vi "RFmx_MeasTest_Analysis.vi"(8 "error in (no error)":errorcluster, 11 "Message_Queues":T3) -> (0 "error out":errorcluster)   [LabVIEW 2014]
uses:
  02_Controls/Message_Queues.ctl
  02_Controls/Message_Data_Ctl.ctl
  15_DataManagement/Analysis_Parameters.ctl
  SubVIs/RFmx_An_Disp_Ctrl.ctl
panel:
  in  "Tab Control":T1=enum."CCDF"
  out "ACP":cluster{"x0":dbl, "dx":dbl, "y":sgl[]}[](graph)=[{"x0"=1134999754.066313, "dx"=998.2196003401557, "y"=array[30055 elements]}, {"x0"=0.0, "dx"=0.0, "y"=[]}, {"x0"=0.0, "dx"=0.0, "y"=[]}, {"x0"=0.0, "dx"=0.0, "y"=[]}, {"x0"=1134999754.066313, "dx"=998.2196003401557, "y"=array[30055 elements]}]
  out "ACP_Data":dbl[](array[numeric])=[750000.0, -20.734813690185547, 53.66733169555664, 3.519465684890747] format="%#_6p"
  out "CHP":cluster{"x0":dbl, "dx":dbl, "y":sgl[]}[](graph)=[{"x0"=1134999754.066313, "dx"=998.2196003401557, "y"=array[30055 elements]}, {"x0"=1134999754.066313, "dx"=998.2196003401557, "y"=array[30055 elements]}]
  out "OBW":cluster{"x0":dbl, "dx":dbl, "y":sgl[]}[](graph)=[{"x0"=1134999754.066313, "dx"=998.2196003401557, "y"=array[30055 elements]}, {"x0"=1134999754.066313, "dx"=998.2196003401557, "y"=array[30055 elements]}]
  out "TXP_PwrTrace":cluster{"x0":dbl, "dx":dbl, "y":sgl[]}(graph)={"x0"=-4.98745570667522e-12, "dx"=1.333333333320651e-05, "y"=[-70.1271, -70.102455, -70.09967, -70.138626, -70.2021, -70.25555, -70.28413, -70.29169, -70.28087, -70.246735, -70.18414, -70.09316, -69.98076, -69.8681, -69.79553, -69.79967, -69.875374, -69.97399, -70.04578, -70.074875, -70.0764, -70.07251, -70.0786, -70.099106, -70.12221, -70.11699, -70.06154, -69.987854, -69.97353, -70.07697, -70.28213, -70.49838, -70.619514, -70.604355, -70.50262, -70.399666, -70.34924, -70.354, -70.3841, -70.40493, -70.39727, -70.36025, -70.31259, -70.28346, -70.279724, -70.2837, -70.28102, -70.27398, -70.273705, -70.28955, -70.32246, -70.36373, -70.40005, -70.4229, -70.43052, -70.42366, -70.40363, -70.3778, -70.36408, -70.38452, -70.44807, -70.549355, -70.66728, -70.747925, -70.71708, -70.54683, -70.28816, -70.03155, -69.85307, -69.78543, -69.80181, -69.82049, -69.76297, -69.637566, -69.54464, -69.58453, -69.76692, -70.01199, -70.22523, -70.36874, -70.46258, -70.54471, -70.628296, -70.689095, -70.6958, -70.644844, -70.56589, -70.49992, -70.466835, -70.457146, -70.45056, -70.43114, -70.392235, -70.34338, -70.30397, -70.285736, -70.28102, -70.272095, -70.249214, -70.227776, -70.24491, -70.31819, -70.41253, -70.4785, -70.50577, -70.51349, -70.51906, -70.53742, -70.59497, -70.73529, -71.00162, -71.38568, -71.789246, -72.070625, -72.15951, -72.077644, -71.88744, -71.65048, -71.38336, -71.0968, -70.85372, -70.712296, -70.648, -70.59169, -70.51985, -70.46071, -70.434654, -70.42709, -70.41435, -70.38291, -70.33717, -70.294846, -70.267975, -70.25562, -70.250694, -70.24638, -70.23686, -70.21681, -70.185425, -70.152855, -70.13762, -70.14813, -70.1704, -70.18109, -70.168976, -70.14167, -70.11527, -70.09345, -70.06084, -70.00988, -69.97303, -70.01334, -70.162346, -70.36518, -70.51255, -70.52762, -70.410835, -70.21521, -70.005104, -69.83721, -69.753, -69.76635, -69.85591, -69.97935, -70.09232, -70.160034, -70.176285, -70.17383, -70.195854, -70.25506, -70.34203, -70.46222, -70.63041, -70.81692, -70.9472, -70.98923, -71.01785, -71.1728, -71.53291, -72.01664, -72.406296, -72.52623, -72.40028, -72.1804, -71.96133, -71.74775, -71.57884, -71.5427, -71.664444, -71.86329, -72.009705, -72.022285, -71.9312, -71.82318, -71.7381, -71.65193, -71.51254, -71.2917, -71.03287, -70.83856, -70.78675, -70.868, -71.01887, -71.202896, -71.43712, -71.73827, -72.08321, -72.42074, -72.6703, -72.712105, -72.46677, -72.00842, -71.53421, -71.24306, -71.24765, -71.53821, -71.9796, -72.376366, -72.59654, -72.640526, -72.58551, -72.46033, -72.21592, -71.82655, -71.36928, -70.96878, -70.70235, -70.57518, -70.55464, -70.60321, -70.671196, -70.69574, -70.64515, -70.55917, -70.52155, -70.60362, -70.83718, -71.20136, -71.60672, -71.91493, -72.01895, -71.92462, -71.7453, -71.60187, -71.52983, -71.46005, -71.2856, -70.983475, -70.640854, -70.35246, -70.154205, -70.0494, -70.03544, -70.094894, -70.19584, -70.31638, -70.43914, -70.52042, -70.50131, -70.36992, -70.1966, -70.08757, -70.114914, -70.280266, -70.516754, -70.73874, -70.904396, -71.013405, -71.041016, -70.93407, -70.69386, -70.42141, -70.24169, -70.20023, -70.24776, -70.31064, -70.36012, -70.392685, -70.38757, -70.330055, -70.24892, -70.188736, -70.15334, -70.11064, -70.04098, -69.960236, -69.90947, -69.93629, -70.0791, -70.33356, -70.624886, -70.83586, -70.89375, -70.814514, -70.66997, -70.5526, -70.55675, -70.7309, -71.01462, -71.242516, -71.27896, -71.148766, -70.98232, -70.870804, -70.81653, -70.76519, -70.67791, -70.57681, -70.49742, -70.42339, -70.31814, -70.21381, -70.21159, -70.38383, -70.68958, -70.97363, -71.07428, -70.959236, -70.73489, -70.52688, -70.393105, -70.333824, -70.32502, -70.33476, -70.33452, -70.309326, -70.263794, -70.22499, -70.22239, -70.25476, -70.29094, -70.30613, -70.300125, -70.29144, -70.30344, -70.35219, -70.433464, -70.51426, -70.549385, -70.519104, -70.44781, -70.38268, -70.35341, -70.35752, -70.38461, -70.448654, -70.590775, -70.83775, -71.13816, -71.36328, -71.40347, -71.26845, -71.06155, -70.86465, -70.68394, -70.50064, -70.32482, -70.18509, -70.09302, -70.034256, -69.9907, -69.96237, -69.96383, -70.00722, -70.1008, -70.25221, -70.43503, -70.563286, -70.54413, -70.37306, -70.14535, -69.97606, -69.93775, -70.051865, -70.298836, -70.63075, -70.96844, -71.191925, -71.19785, -71.00357, -70.74416, -70.549095, -70.45745, -70.44101, -70.46208, -70.487526, -70.48328, -70.42944, -70.336716, -70.23764, -70.16715, -70.15245, -70.20595, -70.33126, -70.523056, -70.75548, -70.97542, -71.127914, -71.20036, -71.23254, -71.283714, -71.37482, -71.45885, -71.4582, -71.33722, -71.131905, -70.918884, -70.764725, -70.68758, -70.66344, -70.66629, -70.69003, -70.72007, -70.712395, -70.63426, -70.510025, -70.401115, -70.349625, -70.3556, -70.38955, -70.41931, -70.42943, -70.419876, -70.392715, -70.3439, -70.26482, -70.16419, -70.09059, -70.11067, -70.25772, -70.50903, -70.78793, -70.98342, -71.03065, -70.987206, -70.957726, -70.95307, -70.904144, -70.802505, -70.74672, -70.8326, -71.03998, -71.23038, -71.261185, -71.11531, -70.89604, -70.718994, -70.64278, -70.67297, -70.77545, -70.88165, -70.92553, -70.91127, -70.90201, -70.920334, -70.9097, -70.81249, -70.642, -70.460976, -70.31799, -70.22179, -70.16339, -70.14114, -70.153564, -70.18681, -70.22244, -70.25476, -70.29089, -70.336296, -70.38193, -70.41022, -70.41077, -70.38516, -70.348206, -70.32399, -70.325325, -70.34256, -70.36334, -70.393364, -70.460625, -70.59186, -70.7767, -70.9539, -71.04438, -71.00727, -70.867874, -70.70291, -70.59369, -70.58453, -70.66925, -70.80333, -70.94123, -71.07266, -71.21135, -71.34671, -71.45471, -71.549774, -71.671684, -71.794785, -71.811935, -71.66149, -71.427444, -71.25798, -71.22795, -71.29315, -71.352036, -71.342224, -71.270226, -71.180084, -71.12189, -71.12526, -71.16607, -71.166954, -71.058426, -70.8422, -70.58765, -70.36951, -70.23198, -70.196075, -70.2832, -70.51522, -70.87754, -71.28055, -71.57588, -71.675446, -71.65345, -71.67442, -71.82185, -72.03004, -72.15217, -72.0683, -71.75293, -71.28349, -70.800285, -70.4402, -70.29247, -70.386894, -70.681244, -71.05052, -71.34525, -71.526794, -71.67786, -71.83254, -71.921036, -71.908615, -71.85493, -71.82098, -71.81082, -71.788025, -71.70886, -71.56084, -71.38074, -71.21522, -71.06775, -70.89776, -70.67848, -70.443886, -70.26495, -70.18929, -70.22381, -70.34598, -70.49758, -70.59422, -70.58327, -70.492256, -70.39598, -70.34745, -70.350945, -70.376526, -70.388756, -70.3667, -70.309906, -70.24661, -70.21888, -70.239075, -70.283875, -70.32356, -70.34142, -70.336464, -70.32062, -70.31242, -70.32254, -70.34507, -70.37217, -70.412254, -70.48494, -70.5921, -70.68931, -70.716415, -70.67915, -70.666595, -70.74049, -70.857124, -70.93891, -70.9912, -71.096535, -71.29889, -71.51818, -71.59646, -71.452415, -71.16241, -70.88185, -70.715324, -70.66288, -70.66028, -70.64644, -70.606415, -70.55378, -70.50803, -70.49969, -70.54775, -70.62311, -70.68454, -70.736206, -70.801315, -70.87974, -70.95877, -71.03975, -71.11876, -71.166214, -71.14653, -71.04972, -70.898445, -70.7247, -70.55195, -70.39522, -70.260086, -70.15135, -70.08678, -70.08174, -70.123795, -70.18848, -70.26684, -70.3716, -70.513985, -70.674736, -70.808716, -70.881485, -70.885155, -70.82721, -70.73247, -70.65466, -70.64117, -70.676765, -70.68882, -70.624115, -70.50197, -70.38329, -70.30879, -70.28491, -70.30879, -70.38329, -70.50113, -70.6197, -70.67169, -70.624115, -70.51857, -70.43616, -70.43359, -70.50927, -70.6081, -70.66765, -70.68427, -70.72201, -70.82337, -70.94429, -71.00236, -70.96122, -70.84161, -70.70359, -70.64045, -70.72783, -70.940865, -71.137505, -71.172806, -71.041145, -70.85834, -70.719444, -70.62562, -70.53578, -70.43355, -70.338165, -70.27004, -70.235825, -70.242905, -70.30614, -70.429855, -70.5876, -70.72852, -70.80606, -70.789406, -70.65997, -70.43023, -70.17071, -69.97722, -69.89921, -69.91674, -69.98164, -70.059425, -70.140335, -70.22925, -70.334366, -70.46442, -70.61354, -70.73899, -70.77561, -70.70575, -70.59821, -70.559265, -70.65948, -70.90869, -71.270645, -71.67924, -72.03883, -72.237366, -72.20009, -71.96115, -71.65437, -71.408066, -71.2635, -71.18208, -71.09467, -70.94478, -70.727875, -70.51102, -70.37953, -70.36407, -70.437836, -70.550835, -70.63729, -70.63367, -70.53299, -70.404144, -70.337685, -70.38474, -70.543526, -70.75984, -70.94081, -71.0143, -70.999954, -70.99277, -71.043396, -71.07776, -70.98049, -70.75311, -70.525215, -70.41042, -70.41771, -70.501976, -70.62645]}
  out "CCDF_PwrTrace":cluster{"x0":dbl, "dx":dbl, "y":sgl[]}[](graph)=[{"x0"=0.0, "dx"=0.05, "y"=[53.66733, 52.4644, 51.195732, 49.906933, 48.5928, 47.24, 45.878, 44.492535, 43.0708, 41.638268, 40.190933, 38.7444, 37.3052, 35.848, 34.410667, 32.9784, 31.523867, 30.067734, 28.628933, 27.1972, 25.780666, 24.380667, 22.984533, 21.613333, 20.296667, 19.015066, 17.751333, 16.544134, 15.362267, 14.232, 13.1368, 12.0996, 11.079866, 10.1244, 9.173734, 8.2868, 7.4492, 6.670533, 5.9525332, 5.295067, 4.6957335, 4.153333, 3.6621332, 3.2249334, 2.8288, 2.4806666, 2.1506667, 1.8712, 1.6233333, 1.4028, 1.2012, 1.028, 0.8810667, 0.74453336, 0.6264, 0.5182667, 0.4148, 0.32906666, 0.2516, 0.18853334, 0.14026667, 0.0992, 0.06893333, 0.048933335, 0.031466667, 0.019066667, 0.010533334, 0.0052, 0.0028, 0.0014666667, 0.0004, 0.0, 0.0, 0.0, 0.0, 0.0, 0.0, 0.0, 0.0, 0.0, 0.0, 0.0, 0.0, 0.0, 0.0, 0.0, 0.0, 0.0, 0.0, 0.0, 0.0, 0.0, 0.0, 0.0, 0.0, 0.0, 0.0, 0.0, 0.0, 0.0, 0.0, 0.0, 0.0, 0.0, 0.0, 0.0, 0.0, 0.0, 0.0, 0.0, 0.0, 0.0, 0.0, 0.0, 0.0, 0.0, 0.0, 0.0, 0.0, 0.0, 0.0, 0.0, 0.0, 0.0, 0.0, 0.0, 0.0, 0.0, 0.0, 0.0, 0.0, 0.0, 0.0, 0.0, 0.0, 0.0, 0.0, 0.0, 0.0, 0.0, 0.0, 0.0, 0.0, 0.0, 0.0, 0.0, 0.0, 0.0, 0.0, 0.0, 0.0, 0.0, 0.0, 0.0, 0.0, 0.0, 0.0, 0.0, 0.0, 0.0, 0.0, 0.0, 0.0, 0.0, 0.0, 0.0, 0.0, 0.0, 0.0, 0.0, 0.0, 0.0, 0.0, 0.0, 0.0, 0.0, 0.0, 0.0, 0.0, 0.0, 0.0, 0.0, 0.0, 0.0, 0.0, 0.0, 0.0, 0.0, 0.0, 0.0, 0.0, 0.0, 0.0, 0.0, 0.0, 0.0, 0.0, 0.0, 0.0, 0.0, 0.0, 0.0, 0.0, 0.0, 0.0, 0.0, 0.0, 0.0, 0.0, 0.0, 0.0, 0.0, 0.0, 0.0, 0.0, 0.0, 0.0, 0.0, 0.0, 0.0, 0.0, 0.0, 0.0, 0.0, 0.0, 0.0, 0.0, 0.0, 0.0, 0.0, 0.0, 0.0, 0.0, 0.0, 0.0, 0.0, 0.0, 0.0, 0.0, 0.0, 0.0, 0.0, 0.0, 0.0, 0.0, 0.0, 0.0, 0.0, 0.0, 0.0, 0.0, 0.0, 0.0, 0.0, 0.0, 0.0, 0.0, 0.0, 0.0, 0.0, 0.0, 0.0, 0.0, 0.0, 0.0, 0.0, 0.0, 0.0, 0.0, 0.0, 0.0, 0.0, 0.0, 0.0, 0.0, 0.0, 0.0, 0.0, 0.0, 0.0, 0.0, 0.0, 0.0, 0.0, 0.0, 0.0, 0.0, 0.0, 0.0, 0.0, 0.0, 0.0, 0.0, 0.0, 0.0, 0.0, 0.0, 0.0, 0.0, 0.0, 0.0, 0.0, 0.0, 0.0, 0.0, 0.0, 0.0, 0.0, 0.0, 0.0, 0.0, 0.0, 0.0, 0.0, 0.0, 0.0, 0.0, 0.0, 0.0, 0.0, 0.0, 0.0, 0.0, 0.0, 0.0, 0.0, 0.0, 0.0, 0.0, 0.0, 0.0, 0.0, 0.0, 0.0, 0.0, 0.0, 0.0, 0.0, 0.0, 0.0, 0.0, 0.0, 0.0, 0.0, 0.0, 0.0, 0.0, 0.0, 0.0, 0.0, 0.0, 0.0, 0.0, 0.0, 0.0, 0.0, 0.0, 0.0, 0.0, 0.0, 0.0, 0.0, 0.0, 0.0, 0.0, 0.0, 0.0, 0.0, 0.0, 0.0, 0.0, 0.0, 0.0, 0.0, 0.0, 0.0, 0.0, 0.0, 0.0, 0.0, 0.0, 0.0, 0.0, 0.0, 0.0, 0.0, 0.0, 0.0, 0.0, 0.0, 0.0, 0.0, 0.0, 0.0, 0.0, 0.0, 0.0, 0.0, 0.0, 0.0]}, {"x0"=0.0, "dx"=0.05, "y"=[36.787945, 36.364418, 35.940945, 35.51759, 35.094402, 34.671444, 34.24878, 33.826458, 33.404545, 32.9831, 32.562187, 32.141865, 31.722195, 31.30324, 30.885061, 30.467726, 30.051294, 29.635832, 29.221403, 28.808071, 28.3959, 27.984957, 27.575306, 27.167011, 26.76014, 26.354755, 25.950926, 25.548716, 25.14819, 24.749414, 24.352455, 23.957375, 23.564243, 23.17312, 22.784075, 22.39717, 22.012466, 21.630032, 21.24993, 20.872221, 20.49697, 20.124235, 19.75408, 19.386568, 19.021753, 18.6597, 18.300467, 17.944107, 17.590683, 17.240246, 16.892855, 16.548563, 16.207422, 15.869487, 15.534806, 15.20343, 14.875409, 14.55079, 14.229618, 13.91194, 13.597798, 13.287235, 12.980292, 12.677009, 12.377422, 12.08157, 11.789486, 11.501204, 11.216754, 10.936168, 10.659473, 10.386697, 10.117864, 9.852996, 9.592114, 9.33524, 9.082389, 8.833577, 8.5888195, 8.348126, 8.111507, 7.8789725, 7.650526, 7.4261727, 7.205915, 6.9897523, 6.7776837, 6.5697045, 6.36581, 6.165992, 5.9702406, 5.778545, 5.590891, 5.4072638, 5.2276454, 5.052017, 4.8803573, 4.7126436, 4.5488515, 4.3889537, 4.232922, 4.0807266, 3.9323359, 3.7877162, 3.6468325, 3.509648, 3.376125, 3.2462234, 3.1199024, 2.997119, 2.8778293, 2.7619884, 2.6495495, 2.540465, 2.4346862, 2.3321629, 2.2328444, 2.1366782, 2.0436118, 1.9535915, 1.8665625, 1.7824696, 1.701257, 1.6228681, 1.5472456, 1.4743322, 1.4040698, 1.3364, 1.2712642, 1.2086037, 1.1483593, 1.0904721, 1.0348829, 0.98153263, 0.9303623, 0.881313, 0.83432627, 0.78934366, 0.7463072, 0.7051592, 0.6658425, 0.62830037, 0.5924767, 0.558316, 0.52576315, 0.49476406, 0.46526518, 0.43721372, 0.4105578, 0.3852463, 0.36122903, 0.3384567, 0.31688094, 0.29645437, 0.2771306, 0.2588643, 0.24161115, 0.22532786, 0.20997226, 0.19550326, 0.18188089, 0.16906624, 0.15702157, 0.14571023, 0.13509673, 0.12514666, 0.11582677, 0.10710493, 0.09895011, 0.09133239, 0.084222965, 0.077594094, 0.071419135, 0.065672494, 0.060329612, 0.055366978, 0.050762083, 0.04649341, 0.042540405, 0.038883466, 0.03550392, 0.032383993, 0.029506788, 0.02685626, 0.0244172, 0.02217519, 0.020116596, 0.018228529, 0.016498832, 0.0149160335, 0.013469341, 0.012148602, 0.010944282, 0.009847437, 0.008849691, 0.007943204, 0.007120654, 0.0063752076, 0.0057004965, 0.005090594, 0.004539993, 0.004043582, 0.0035966237, 0.003194734, 0.0028338607, 0.0025102647, 0.0022205, 0.0019613956, 0.0017300382, 0.0015237544, 0.0013400955, 0.0011768217, 0.0010318871, 0.0009034264, 0.0007897411, 0.0006892875, 0.0006006644, 0.0005226023, 0.0004539527, 0.00039367852, 0.0003408446, 0.00029460926, 0.00025421623, 0.00021898713, 0.00018831449, 0.00016165532, 0.00013852515, 0.00011849246, 0.000101173624, 8.622819e-05, 7.3354604e-05, 6.228628e-05, 5.2787957e-05, 4.4652443e-05, 3.7697617e-05, 3.1763702e-05, 2.6710808e-05, 2.2416698e-05, 1.8774781e-05, 1.5692298e-05, 1.3088694e-05, 1.08941595e-05, 9.048326e-06, 7.4991e-06, 6.201627e-06, 5.1173697e-06, 4.2132915e-06, 3.461136e-06, 2.836788e-06, 2.3197156e-06, 1.8924771e-06, 1.5402914e-06, 1.250661e-06, 1.0130451e-06, 8.185747e-07, 6.598055e-07, 5.3050474e-07, 4.254668e-07, 3.4035529e-07, 2.7156693e-07, 2.1611548e-07, 1.7153243e-07, 1.357828e-07, 1.0719338e-07, 8.439218e-08, 6.62573e-08, 5.1873865e-08, 4.0497927e-08, 3.1526227e-08, 2.4471005e-08, 1.8939026e-08, 1.461419e-08, 1.1243155e-08, 8.623487e-09, 6.593919e-09, 5.0263744e-09, 3.8194514e-09, 2.8931189e-09, 2.1844124e-09, 1.6439551e-09, 1.2331498e-09, 9.2192537e-10, 6.8693073e-10, 5.1009436e-10, 3.7747766e-10, 2.7836708e-10, 2.045563e-10, 1.497816e-10, 1.09279e-10, 7.943822e-11, 5.753319e-11, 4.151308e-11, 2.984079e-11, 2.136857e-11, 1.5242675e-11, 1.08304875e-11, 7.6650734e-12, 5.4031393e-12, 3.7933025e-12, 2.6522215e-12, 1.8467268e-12, 1.2804867e-12, 8.8410946e-13, 6.0781897e-13, 4.1606207e-13, 2.8355402e-13, 1.9239123e-13, 1.2995236e-13, 8.737957e-14, 5.848435e-14, 3.896281e-14, 2.5835592e-14, 1.7049845e-14, 1.1197791e-14, 7.318634e-15, 4.7598025e-15, 3.0802383e-15, 1.9833124e-15, 1.2705274e-15, 8.097247e-16, 5.133638e-16, 3.2375868e-16, 2.0309505e-16, 1.267162e-16, 7.86308e-17, 4.852366e-17, 2.9777407e-17, 1.8170405e-17, 1.10244845e-17, 6.650268e-18, 3.9882104e-18, 2.3776376e-18, 1.4090037e-18, 8.2994133e-19, 4.8587095e-19, 2.8268445e-19, 1.6344032e-19, 9.389906e-20, 5.36014e-20, 3.039986e-20, 1.7128329e-20, 9.586792e-21, 5.329827e-21, 2.94307e-21, 1.6139929e-21, 8.789851e-22, 4.753412e-22, 2.552336e-22, 1.3606395e-22, 7.200868e-23, 3.7829146e-23, 1.972564e-23, 1.0208479e-23, 5.242983e-24, 2.6720525e-24, 1.3512067e-24, 6.779063e-25, 3.3740296e-25, 1.6657864e-25, 8.157184e-26, 3.9616006e-26, 1.9079589e-26, 9.111568e-27, 4.314202e-27, 2.0251076e-27, 9.423071e-28, 4.345997e-28, 1.9865274e-28, 8.998346e-29, 4.0387624e-29, 1.7959954e-29, 7.9120106e-30, 3.452598e-30, 1.4922271e-30, 6.387123e-31, 2.707125e-31, 1.1360423e-31, 4.7196953e-32, 1.9409576e-32, 7.900411e-33, 3.182461e-33, 1.2685392e-33, 5.00287e-34, 1.9518905e-34, 7.532834e-35, 2.8752345e-35, 1.08528714e-35, 4.0505728e-36, 1.4946238e-36, 5.451721e-37, 1.965457e-37, 7.002659e-38, 2.4653156e-38, 8.574959e-39, 2.946325e-39, 9.99901e-40, 3.35119e-40, 1.10903e-40, 3.62348e-41, 1.16868e-41]}]
  out "CCDF_Data":dbl[](array[numeric])=[750000.0, -20.734813690185547, 53.66733333333333, 3.519465684890747] format="%#_6p"
  out "Spectrum":cluster{"x0":dbl, "dx":dbl, "y":sgl[]}(graph)={"x0"=-4.98745570667522e-12, "dx"=1.333333333320651e-05, "y"=[-70.1271, -70.102455, -70.09967, -70.138626, -70.2021, -70.25555, -70.28413, -70.29169, -70.28087, -70.246735, -70.18414, -70.09316, -69.98076, -69.8681, -69.79553, -69.79967, -69.875374, -69.97399, -70.04578, -70.074875, -70.0764, -70.07251, -70.0786, -70.099106, -70.12221, -70.11699, -70.06154, -69.987854, -69.97353, -70.07697, -70.28213, -70.49838, -70.619514, -70.604355, -70.50262, -70.399666, -70.34924, -70.354, -70.3841, -70.40493, -70.39727, -70.36025, -70.31259, -70.28346, -70.279724, -70.2837, -70.28102, -70.27398, -70.273705, -70.28955, -70.32246, -70.36373, -70.40005, -70.4229, -70.43052, -70.42366, -70.40363, -70.3778, -70.36408, -70.38452, -70.44807, -70.549355, -70.66728, -70.747925, -70.71708, -70.54683, -70.28816, -70.03155, -69.85307, -69.78543, -69.80181, -69.82049, -69.76297, -69.637566, -69.54464, -69.58453, -69.76692, -70.01199, -70.22523, -70.36874, -70.46258, -70.54471, -70.628296, -70.689095, -70.6958, -70.644844, -70.56589, -70.49992, -70.466835, -70.457146, -70.45056, -70.43114, -70.392235, -70.34338, -70.30397, -70.285736, -70.28102, -70.272095, -70.249214, -70.227776, -70.24491, -70.31819, -70.41253, -70.4785, -70.50577, -70.51349, -70.51906, -70.53742, -70.59497, -70.73529, -71.00162, -71.38568, -71.789246, -72.070625, -72.15951, -72.077644, -71.88744, -71.65048, -71.38336, -71.0968, -70.85372, -70.712296, -70.648, -70.59169, -70.51985, -70.46071, -70.434654, -70.42709, -70.41435, -70.38291, -70.33717, -70.294846, -70.267975, -70.25562, -70.250694, -70.24638, -70.23686, -70.21681, -70.185425, -70.152855, -70.13762, -70.14813, -70.1704, -70.18109, -70.168976, -70.14167, -70.11527, -70.09345, -70.06084, -70.00988, -69.97303, -70.01334, -70.162346, -70.36518, -70.51255, -70.52762, -70.410835, -70.21521, -70.005104, -69.83721, -69.753, -69.76635, -69.85591, -69.97935, -70.09232, -70.160034, -70.176285, -70.17383, -70.195854, -70.25506, -70.34203, -70.46222, -70.63041, -70.81692, -70.9472, -70.98923, -71.01785, -71.1728, -71.53291, -72.01664, -72.406296, -72.52623, -72.40028, -72.1804, -71.96133, -71.74775, -71.57884, -71.5427, -71.664444, -71.86329, -72.009705, -72.022285, -71.9312, -71.82318, -71.7381, -71.65193, -71.51254, -71.2917, -71.03287, -70.83856, -70.78675, -70.868, -71.01887, -71.202896, -71.43712, -71.73827, -72.08321, -72.42074, -72.6703, -72.712105, -72.46677, -72.00842, -71.53421, -71.24306, -71.24765, -71.53821, -71.9796, -72.376366, -72.59654, -72.640526, -72.58551, -72.46033, -72.21592, -71.82655, -71.36928, -70.96878, -70.70235, -70.57518, -70.55464, -70.60321, -70.671196, -70.69574, -70.64515, -70.55917, -70.52155, -70.60362, -70.83718, -71.20136, -71.60672, -71.91493, -72.01895, -71.92462, -71.7453, -71.60187, -71.52983, -71.46005, -71.2856, -70.983475, -70.640854, -70.35246, -70.154205, -70.0494, -70.03544, -70.094894, -70.19584, -70.31638, -70.43914, -70.52042, -70.50131, -70.36992, -70.1966, -70.08757, -70.114914, -70.280266, -70.516754, -70.73874, -70.904396, -71.013405, -71.041016, -70.93407, -70.69386, -70.42141, -70.24169, -70.20023, -70.24776, -70.31064, -70.36012, -70.392685, -70.38757, -70.330055, -70.24892, -70.188736, -70.15334, -70.11064, -70.04098, -69.960236, -69.90947, -69.93629, -70.0791, -70.33356, -70.624886, -70.83586, -70.89375, -70.814514, -70.66997, -70.5526, -70.55675, -70.7309, -71.01462, -71.242516, -71.27896, -71.148766, -70.98232, -70.870804, -70.81653, -70.76519, -70.67791, -70.57681, -70.49742, -70.42339, -70.31814, -70.21381, -70.21159, -70.38383, -70.68958, -70.97363, -71.07428, -70.959236, -70.73489, -70.52688, -70.393105, -70.333824, -70.32502, -70.33476, -70.33452, -70.309326, -70.263794, -70.22499, -70.22239, -70.25476, -70.29094, -70.30613, -70.300125, -70.29144, -70.30344, -70.35219, -70.433464, -70.51426, -70.549385, -70.519104, -70.44781, -70.38268, -70.35341, -70.35752, -70.38461, -70.448654, -70.590775, -70.83775, -71.13816, -71.36328, -71.40347, -71.26845, -71.06155, -70.86465, -70.68394, -70.50064, -70.32482, -70.18509, -70.09302, -70.034256, -69.9907, -69.96237, -69.96383, -70.00722, -70.1008, -70.25221, -70.43503, -70.563286, -70.54413, -70.37306, -70.14535, -69.97606, -69.93775, -70.051865, -70.298836, -70.63075, -70.96844, -71.191925, -71.19785, -71.00357, -70.74416, -70.549095, -70.45745, -70.44101, -70.46208, -70.487526, -70.48328, -70.42944, -70.336716, -70.23764, -70.16715, -70.15245, -70.20595, -70.33126, -70.523056, -70.75548, -70.97542, -71.127914, -71.20036, -71.23254, -71.283714, -71.37482, -71.45885, -71.4582, -71.33722, -71.131905, -70.918884, -70.764725, -70.68758, -70.66344, -70.66629, -70.69003, -70.72007, -70.712395, -70.63426, -70.510025, -70.401115, -70.349625, -70.3556, -70.38955, -70.41931, -70.42943, -70.419876, -70.392715, -70.3439, -70.26482, -70.16419, -70.09059, -70.11067, -70.25772, -70.50903, -70.78793, -70.98342, -71.03065, -70.987206, -70.957726, -70.95307, -70.904144, -70.802505, -70.74672, -70.8326, -71.03998, -71.23038, -71.261185, -71.11531, -70.89604, -70.718994, -70.64278, -70.67297, -70.77545, -70.88165, -70.92553, -70.91127, -70.90201, -70.920334, -70.9097, -70.81249, -70.642, -70.460976, -70.31799, -70.22179, -70.16339, -70.14114, -70.153564, -70.18681, -70.22244, -70.25476, -70.29089, -70.336296, -70.38193, -70.41022, -70.41077, -70.38516, -70.348206, -70.32399, -70.325325, -70.34256, -70.36334, -70.393364, -70.460625, -70.59186, -70.7767, -70.9539, -71.04438, -71.00727, -70.867874, -70.70291, -70.59369, -70.58453, -70.66925, -70.80333, -70.94123, -71.07266, -71.21135, -71.34671, -71.45471, -71.549774, -71.671684, -71.794785, -71.811935, -71.66149, -71.427444, -71.25798, -71.22795, -71.29315, -71.352036, -71.342224, -71.270226, -71.180084, -71.12189, -71.12526, -71.16607, -71.166954, -71.058426, -70.8422, -70.58765, -70.36951, -70.23198, -70.196075, -70.2832, -70.51522, -70.87754, -71.28055, -71.57588, -71.675446, -71.65345, -71.67442, -71.82185, -72.03004, -72.15217, -72.0683, -71.75293, -71.28349, -70.800285, -70.4402, -70.29247, -70.386894, -70.681244, -71.05052, -71.34525, -71.526794, -71.67786, -71.83254, -71.921036, -71.908615, -71.85493, -71.82098, -71.81082, -71.788025, -71.70886, -71.56084, -71.38074, -71.21522, -71.06775, -70.89776, -70.67848, -70.443886, -70.26495, -70.18929, -70.22381, -70.34598, -70.49758, -70.59422, -70.58327, -70.492256, -70.39598, -70.34745, -70.350945, -70.376526, -70.388756, -70.3667, -70.309906, -70.24661, -70.21888, -70.239075, -70.283875, -70.32356, -70.34142, -70.336464, -70.32062, -70.31242, -70.32254, -70.34507, -70.37217, -70.412254, -70.48494, -70.5921, -70.68931, -70.716415, -70.67915, -70.666595, -70.74049, -70.857124, -70.93891, -70.9912, -71.096535, -71.29889, -71.51818, -71.59646, -71.452415, -71.16241, -70.88185, -70.715324, -70.66288, -70.66028, -70.64644, -70.606415, -70.55378, -70.50803, -70.49969, -70.54775, -70.62311, -70.68454, -70.736206, -70.801315, -70.87974, -70.95877, -71.03975, -71.11876, -71.166214, -71.14653, -71.04972, -70.898445, -70.7247, -70.55195, -70.39522, -70.260086, -70.15135, -70.08678, -70.08174, -70.123795, -70.18848, -70.26684, -70.3716, -70.513985, -70.674736, -70.808716, -70.881485, -70.885155, -70.82721, -70.73247, -70.65466, -70.64117, -70.676765, -70.68882, -70.624115, -70.50197, -70.38329, -70.30879, -70.28491, -70.30879, -70.38329, -70.50113, -70.6197, -70.67169, -70.624115, -70.51857, -70.43616, -70.43359, -70.50927, -70.6081, -70.66765, -70.68427, -70.72201, -70.82337, -70.94429, -71.00236, -70.96122, -70.84161, -70.70359, -70.64045, -70.72783, -70.940865, -71.137505, -71.172806, -71.041145, -70.85834, -70.719444, -70.62562, -70.53578, -70.43355, -70.338165, -70.27004, -70.235825, -70.242905, -70.30614, -70.429855, -70.5876, -70.72852, -70.80606, -70.789406, -70.65997, -70.43023, -70.17071, -69.97722, -69.89921, -69.91674, -69.98164, -70.059425, -70.140335, -70.22925, -70.334366, -70.46442, -70.61354, -70.73899, -70.77561, -70.70575, -70.59821, -70.559265, -70.65948, -70.90869, -71.270645, -71.67924, -72.03883, -72.237366, -72.20009, -71.96115, -71.65437, -71.408066, -71.2635, -71.18208, -71.09467, -70.94478, -70.727875, -70.51102, -70.37953, -70.36407, -70.437836, -70.550835, -70.63729, -70.63367, -70.53299, -70.404144, -70.337685, -70.38474, -70.543526, -70.75984, -70.94081, -71.0143, -70.999954, -70.99277, -71.043396, -71.07776, -70.98049, -70.75311, -70.525215, -70.41042, -70.41771, -70.501976, -70.62645]}
  out "Spectrum_Data":dbl[](array[numeric])=[750000.0, -20.734813690185547, 53.66733333333333, 3.519465684890747] format="%#_6p"
  out "IQ_Data":cluster{"x0":dbl, "dx":dbl, "y":sgl[]}(graph)={"x0"=-4.98745570667522e-12, "dx"=1.333333333320651e-05, "y"=[-70.1271, -70.102455, -70.09967, -70.138626, -70.2021, -70.25555, -70.28413, -70.29169, -70.28087, -70.246735, -70.18414, -70.09316, -69.98076, -69.8681, -69.79553, -69.79967, -69.875374, -69.97399, -70.04578, -70.074875, -70.0764, -70.07251, -70.0786, -70.099106, -70.12221, -70.11699, -70.06154, -69.987854, -69.97353, -70.07697, -70.28213, -70.49838, -70.619514, -70.604355, -70.50262, -70.399666, -70.34924, -70.354, -70.3841, -70.40493, -70.39727, -70.36025, -70.31259, -70.28346, -70.279724, -70.2837, -70.28102, -70.27398, -70.273705, -70.28955, -70.32246, -70.36373, -70.40005, -70.4229, -70.43052, -70.42366, -70.40363, -70.3778, -70.36408, -70.38452, -70.44807, -70.549355, -70.66728, -70.747925, -70.71708, -70.54683, -70.28816, -70.03155, -69.85307, -69.78543, -69.80181, -69.82049, -69.76297, -69.637566, -69.54464, -69.58453, -69.76692, -70.01199, -70.22523, -70.36874, -70.46258, -70.54471, -70.628296, -70.689095, -70.6958, -70.644844, -70.56589, -70.49992, -70.466835, -70.457146, -70.45056, -70.43114, -70.392235, -70.34338, -70.30397, -70.285736, -70.28102, -70.272095, -70.249214, -70.227776, -70.24491, -70.31819, -70.41253, -70.4785, -70.50577, -70.51349, -70.51906, -70.53742, -70.59497, -70.73529, -71.00162, -71.38568, -71.789246, -72.070625, -72.15951, -72.077644, -71.88744, -71.65048, -71.38336, -71.0968, -70.85372, -70.712296, -70.648, -70.59169, -70.51985, -70.46071, -70.434654, -70.42709, -70.41435, -70.38291, -70.33717, -70.294846, -70.267975, -70.25562, -70.250694, -70.24638, -70.23686, -70.21681, -70.185425, -70.152855, -70.13762, -70.14813, -70.1704, -70.18109, -70.168976, -70.14167, -70.11527, -70.09345, -70.06084, -70.00988, -69.97303, -70.01334, -70.162346, -70.36518, -70.51255, -70.52762, -70.410835, -70.21521, -70.005104, -69.83721, -69.753, -69.76635, -69.85591, -69.97935, -70.09232, -70.160034, -70.176285, -70.17383, -70.195854, -70.25506, -70.34203, -70.46222, -70.63041, -70.81692, -70.9472, -70.98923, -71.01785, -71.1728, -71.53291, -72.01664, -72.406296, -72.52623, -72.40028, -72.1804, -71.96133, -71.74775, -71.57884, -71.5427, -71.664444, -71.86329, -72.009705, -72.022285, -71.9312, -71.82318, -71.7381, -71.65193, -71.51254, -71.2917, -71.03287, -70.83856, -70.78675, -70.868, -71.01887, -71.202896, -71.43712, -71.73827, -72.08321, -72.42074, -72.6703, -72.712105, -72.46677, -72.00842, -71.53421, -71.24306, -71.24765, -71.53821, -71.9796, -72.376366, -72.59654, -72.640526, -72.58551, -72.46033, -72.21592, -71.82655, -71.36928, -70.96878, -70.70235, -70.57518, -70.55464, -70.60321, -70.671196, -70.69574, -70.64515, -70.55917, -70.52155, -70.60362, -70.83718, -71.20136, -71.60672, -71.91493, -72.01895, -71.92462, -71.7453, -71.60187, -71.52983, -71.46005, -71.2856, -70.983475, -70.640854, -70.35246, -70.154205, -70.0494, -70.03544, -70.094894, -70.19584, -70.31638, -70.43914, -70.52042, -70.50131, -70.36992, -70.1966, -70.08757, -70.114914, -70.280266, -70.516754, -70.73874, -70.904396, -71.013405, -71.041016, -70.93407, -70.69386, -70.42141, -70.24169, -70.20023, -70.24776, -70.31064, -70.36012, -70.392685, -70.38757, -70.330055, -70.24892, -70.188736, -70.15334, -70.11064, -70.04098, -69.960236, -69.90947, -69.93629, -70.0791, -70.33356, -70.624886, -70.83586, -70.89375, -70.814514, -70.66997, -70.5526, -70.55675, -70.7309, -71.01462, -71.242516, -71.27896, -71.148766, -70.98232, -70.870804, -70.81653, -70.76519, -70.67791, -70.57681, -70.49742, -70.42339, -70.31814, -70.21381, -70.21159, -70.38383, -70.68958, -70.97363, -71.07428, -70.959236, -70.73489, -70.52688, -70.393105, -70.333824, -70.32502, -70.33476, -70.33452, -70.309326, -70.263794, -70.22499, -70.22239, -70.25476, -70.29094, -70.30613, -70.300125, -70.29144, -70.30344, -70.35219, -70.433464, -70.51426, -70.549385, -70.519104, -70.44781, -70.38268, -70.35341, -70.35752, -70.38461, -70.448654, -70.590775, -70.83775, -71.13816, -71.36328, -71.40347, -71.26845, -71.06155, -70.86465, -70.68394, -70.50064, -70.32482, -70.18509, -70.09302, -70.034256, -69.9907, -69.96237, -69.96383, -70.00722, -70.1008, -70.25221, -70.43503, -70.563286, -70.54413, -70.37306, -70.14535, -69.97606, -69.93775, -70.051865, -70.298836, -70.63075, -70.96844, -71.191925, -71.19785, -71.00357, -70.74416, -70.549095, -70.45745, -70.44101, -70.46208, -70.487526, -70.48328, -70.42944, -70.336716, -70.23764, -70.16715, -70.15245, -70.20595, -70.33126, -70.523056, -70.75548, -70.97542, -71.127914, -71.20036, -71.23254, -71.283714, -71.37482, -71.45885, -71.4582, -71.33722, -71.131905, -70.918884, -70.764725, -70.68758, -70.66344, -70.66629, -70.69003, -70.72007, -70.712395, -70.63426, -70.510025, -70.401115, -70.349625, -70.3556, -70.38955, -70.41931, -70.42943, -70.419876, -70.392715, -70.3439, -70.26482, -70.16419, -70.09059, -70.11067, -70.25772, -70.50903, -70.78793, -70.98342, -71.03065, -70.987206, -70.957726, -70.95307, -70.904144, -70.802505, -70.74672, -70.8326, -71.03998, -71.23038, -71.261185, -71.11531, -70.89604, -70.718994, -70.64278, -70.67297, -70.77545, -70.88165, -70.92553, -70.91127, -70.90201, -70.920334, -70.9097, -70.81249, -70.642, -70.460976, -70.31799, -70.22179, -70.16339, -70.14114, -70.153564, -70.18681, -70.22244, -70.25476, -70.29089, -70.336296, -70.38193, -70.41022, -70.41077, -70.38516, -70.348206, -70.32399, -70.325325, -70.34256, -70.36334, -70.393364, -70.460625, -70.59186, -70.7767, -70.9539, -71.04438, -71.00727, -70.867874, -70.70291, -70.59369, -70.58453, -70.66925, -70.80333, -70.94123, -71.07266, -71.21135, -71.34671, -71.45471, -71.549774, -71.671684, -71.794785, -71.811935, -71.66149, -71.427444, -71.25798, -71.22795, -71.29315, -71.352036, -71.342224, -71.270226, -71.180084, -71.12189, -71.12526, -71.16607, -71.166954, -71.058426, -70.8422, -70.58765, -70.36951, -70.23198, -70.196075, -70.2832, -70.51522, -70.87754, -71.28055, -71.57588, -71.675446, -71.65345, -71.67442, -71.82185, -72.03004, -72.15217, -72.0683, -71.75293, -71.28349, -70.800285, -70.4402, -70.29247, -70.386894, -70.681244, -71.05052, -71.34525, -71.526794, -71.67786, -71.83254, -71.921036, -71.908615, -71.85493, -71.82098, -71.81082, -71.788025, -71.70886, -71.56084, -71.38074, -71.21522, -71.06775, -70.89776, -70.67848, -70.443886, -70.26495, -70.18929, -70.22381, -70.34598, -70.49758, -70.59422, -70.58327, -70.492256, -70.39598, -70.34745, -70.350945, -70.376526, -70.388756, -70.3667, -70.309906, -70.24661, -70.21888, -70.239075, -70.283875, -70.32356, -70.34142, -70.336464, -70.32062, -70.31242, -70.32254, -70.34507, -70.37217, -70.412254, -70.48494, -70.5921, -70.68931, -70.716415, -70.67915, -70.666595, -70.74049, -70.857124, -70.93891, -70.9912, -71.096535, -71.29889, -71.51818, -71.59646, -71.452415, -71.16241, -70.88185, -70.715324, -70.66288, -70.66028, -70.64644, -70.606415, -70.55378, -70.50803, -70.49969, -70.54775, -70.62311, -70.68454, -70.736206, -70.801315, -70.87974, -70.95877, -71.03975, -71.11876, -71.166214, -71.14653, -71.04972, -70.898445, -70.7247, -70.55195, -70.39522, -70.260086, -70.15135, -70.08678, -70.08174, -70.123795, -70.18848, -70.26684, -70.3716, -70.513985, -70.674736, -70.808716, -70.881485, -70.885155, -70.82721, -70.73247, -70.65466, -70.64117, -70.676765, -70.68882, -70.624115, -70.50197, -70.38329, -70.30879, -70.28491, -70.30879, -70.38329, -70.50113, -70.6197, -70.67169, -70.624115, -70.51857, -70.43616, -70.43359, -70.50927, -70.6081, -70.66765, -70.68427, -70.72201, -70.82337, -70.94429, -71.00236, -70.96122, -70.84161, -70.70359, -70.64045, -70.72783, -70.940865, -71.137505, -71.172806, -71.041145, -70.85834, -70.719444, -70.62562, -70.53578, -70.43355, -70.338165, -70.27004, -70.235825, -70.242905, -70.30614, -70.429855, -70.5876, -70.72852, -70.80606, -70.789406, -70.65997, -70.43023, -70.17071, -69.97722, -69.89921, -69.91674, -69.98164, -70.059425, -70.140335, -70.22925, -70.334366, -70.46442, -70.61354, -70.73899, -70.77561, -70.70575, -70.59821, -70.559265, -70.65948, -70.90869, -71.270645, -71.67924, -72.03883, -72.237366, -72.20009, -71.96115, -71.65437, -71.408066, -71.2635, -71.18208, -71.09467, -70.94478, -70.727875, -70.51102, -70.37953, -70.36407, -70.437836, -70.550835, -70.63729, -70.63367, -70.53299, -70.404144, -70.337685, -70.38474, -70.543526, -70.75984, -70.94081, -71.0143, -70.999954, -70.99277, -71.043396, -71.07776, -70.98049, -70.75311, -70.525215, -70.41042, -70.41771, -70.501976, -70.62645]}
  out "PeakPwrs_Data":sgl[](array[numeric])=[750000.0, -20.734814, 53.66733, 3.5194657] format="%#_6p"
  out "IMD_Spectrum":cluster{"x0":dbl, "dx":dbl, "y":sgl[]}[](graph)
  out "SFDR_Spectrum":cluster{"x0":dbl, "dx":dbl, "y":sgl[]}[](graph)
  out "PeakPwrs_Data 2":sgl[](array[numeric])=[750000.0, -20.734814, 53.66733, 3.5194657] format="%#_6p"
  out "PeakPwrs_Data 3":dbl[](array[numeric])=[750000.0, -20.734813690185547, 53.66733169555664, 3.519465684890747] format="%#_6p"
  out "Harmonics_Spectrum":cluster{"x0":dbl, "dx":dbl, "y":sgl[]}[](graph)
  in  "Analysis_Parameters":T2={"carrier frequency"=1150000000.0, "IQ rate (S/s)"=0.0, "samples per record"=0, "Signal Bandwidth (Hz)"=30000000.0, "Resolution Bandwidth (Hz)"=0.0, "Ref ch Bandwidth (Hz)"=3840000.0, "Offset_Freq(Hz)"=[10000000.0, 7500000.0, 12500000.0], "Integration_Bandwidth(Hz)"=[9000000.0, 3840000.0, 3840000.0]} {"Ref ch Bandwidth (Hz)" format="%#_6p"; "Integration_Bandwidth(Hz)" format="%#_6p"; "Offset_Freq(Hz)" format="%#_6p"; "Resolution Bandwidth (Hz)" format="%#_6p"; "Signal Bandwidth (Hz)" format="%#_6p"; "IQ rate (S/s)" format="%#_6p"; "carrier frequency" format="%#_6p"}
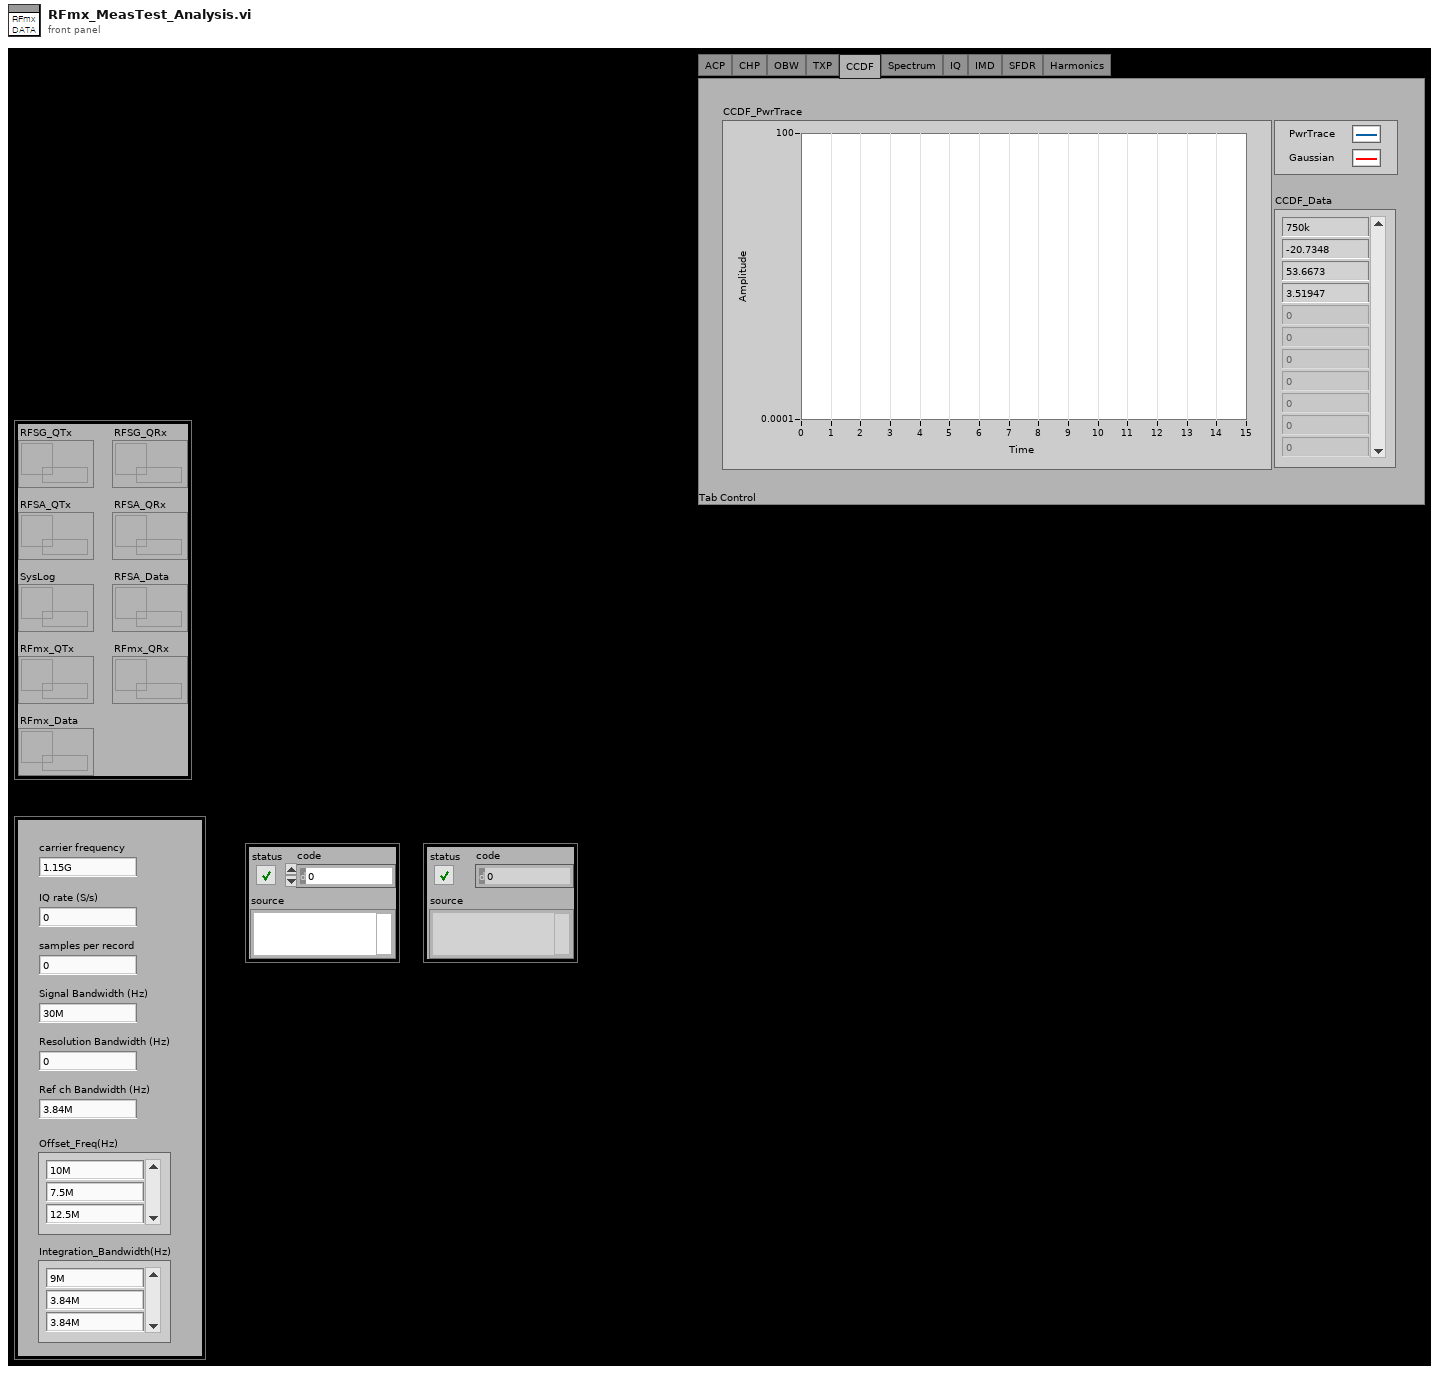
[diagram p1: front panel]
types:
  T1 = typedef "RFmx_An_Disp_Ctrl.ctl" = enum32{"ACP", "CHP", "OBW", "TXP", "CCDF", "Spectrum", "IQ", "IMD", "SFDR", "Harmonics"}
  T2 = typedef "Analysis_Parameters.ctl" = cluster{"carrier frequency":dbl, "IQ rate (S/s)":dbl, "samples per record":i64, "Signal Bandwidth (Hz)":dbl, "Resolution Bandwidth (Hz)":dbl, "Ref ch Bandwidth (Hz)":dbl, "Offset_Freq(Hz)":dbl[], "Integration_Bandwidth(Hz)":dbl[]}
  T3 = typedef "Message_Queues.ctl" = cluster{"RFSG_QTx":refnum<queue>, "RFSG_QRx":refnum<queue>, "RFSA_QTx":refnum<queue>, "RFSA_QRx":refnum<queue>, "SysLog":refnum<queue>, "RFSA_Data":refnum<queue>, "RFmx_QTx":refnum<queue>, "RFmx_QRx":refnum<queue>, "RFmx_Data":refnum<queue>}
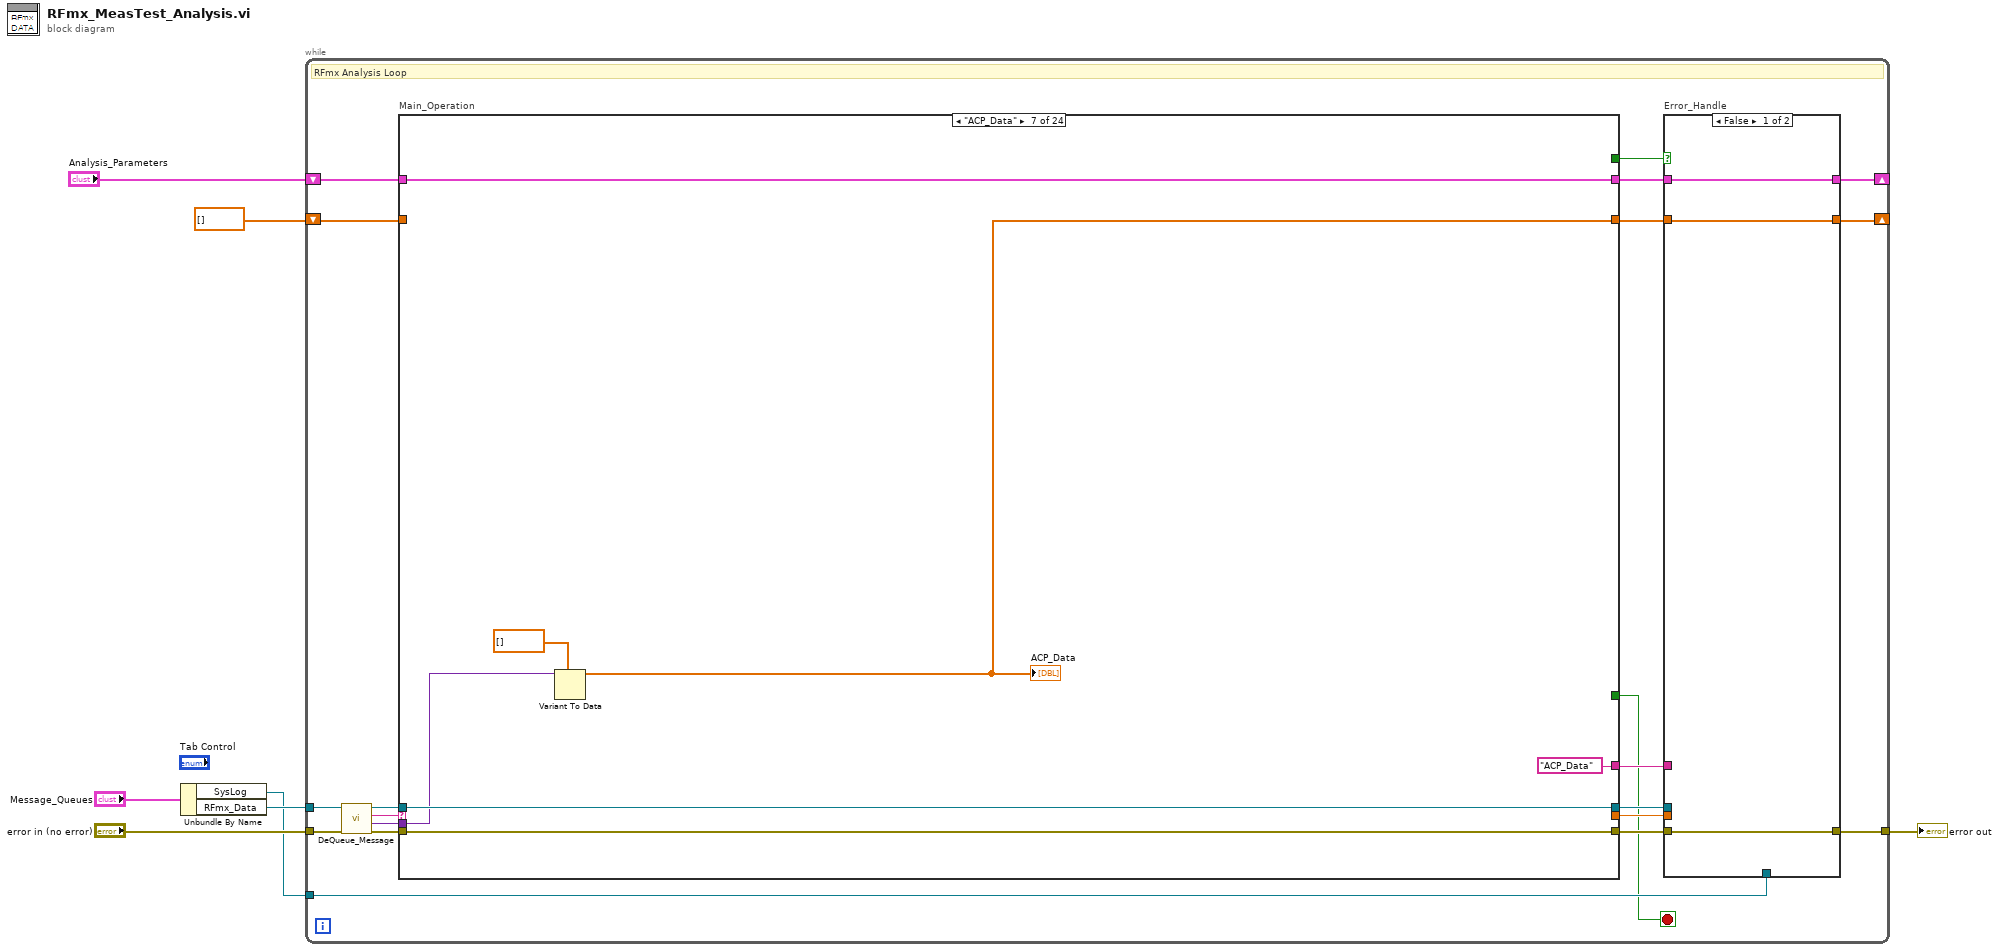
[diagram p0: block diagram]
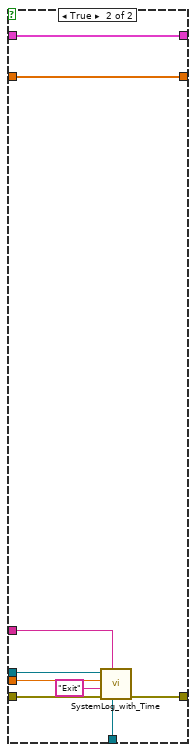
[diagram p2: hidden frame]
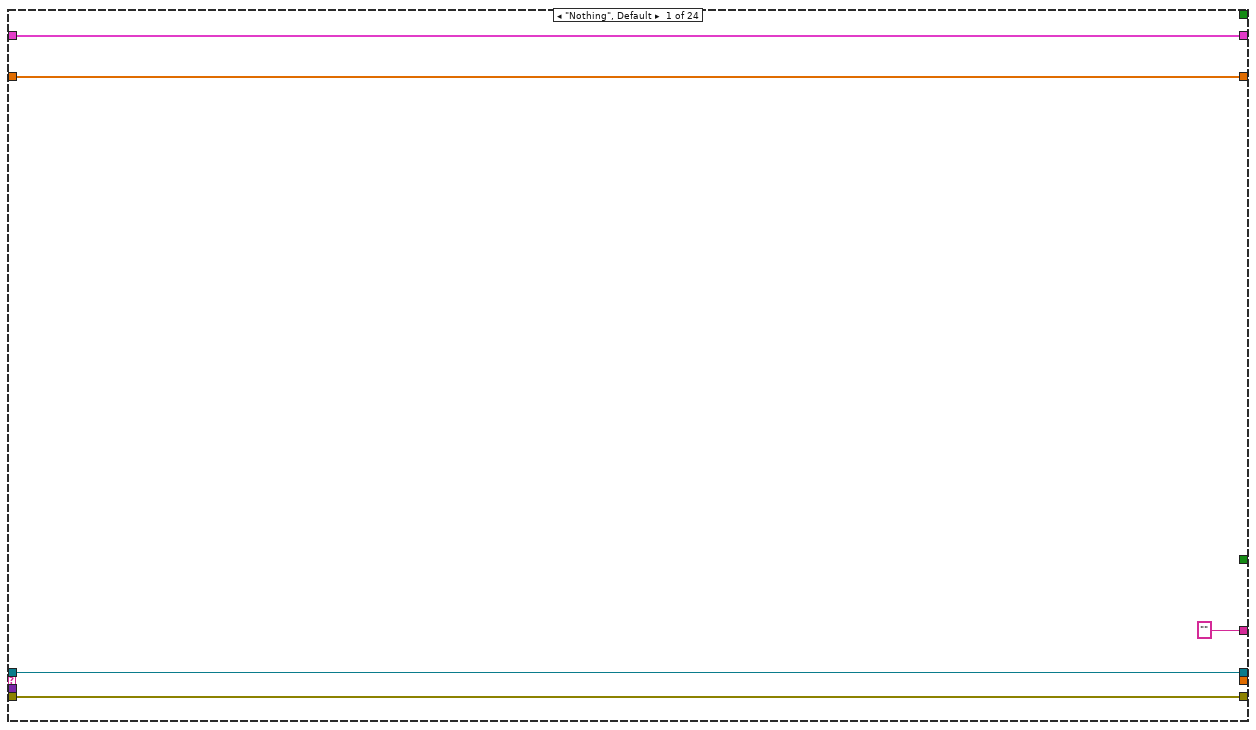
[diagram p3: hidden frame]
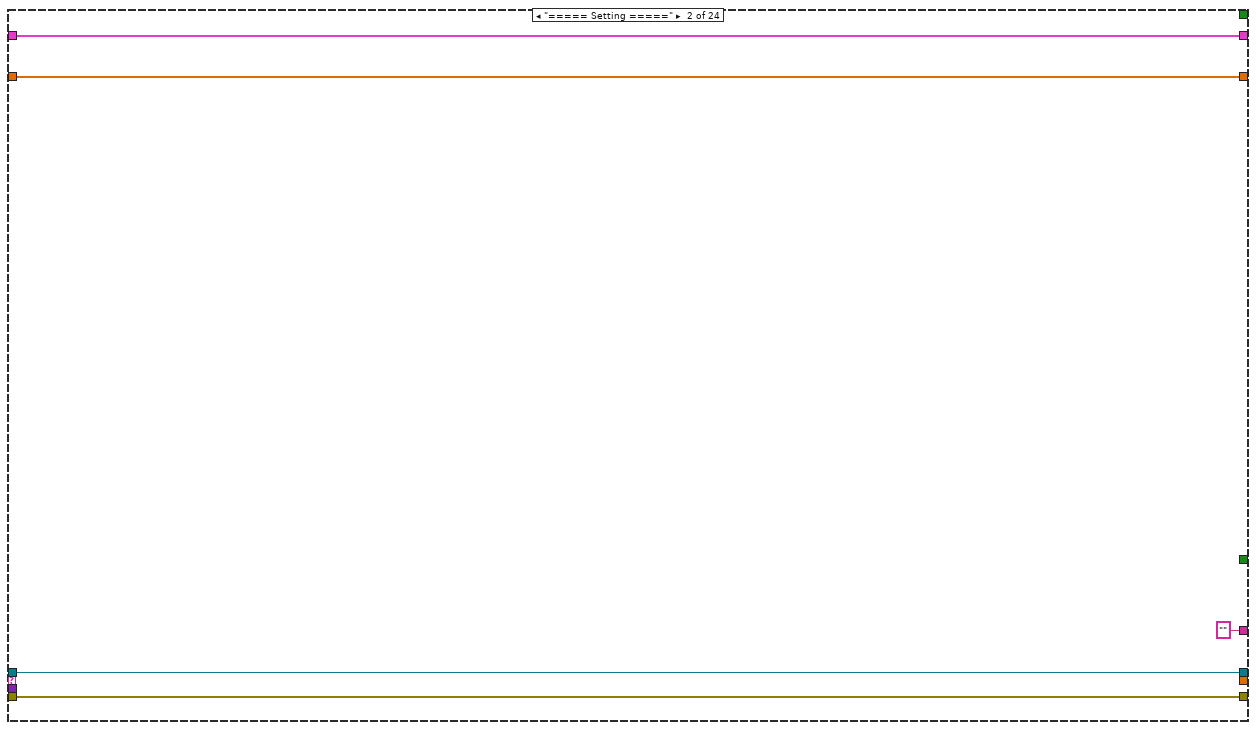
[diagram p4: hidden frame]
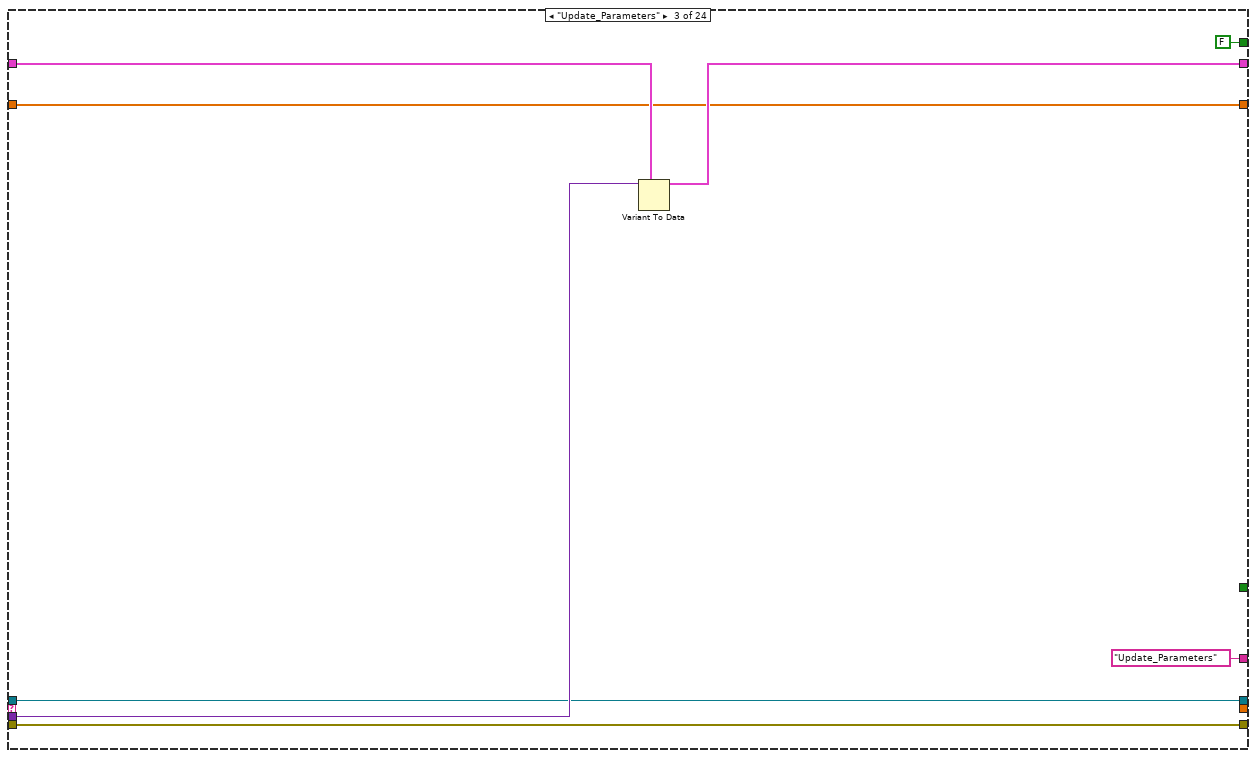
[diagram p5: hidden frame]
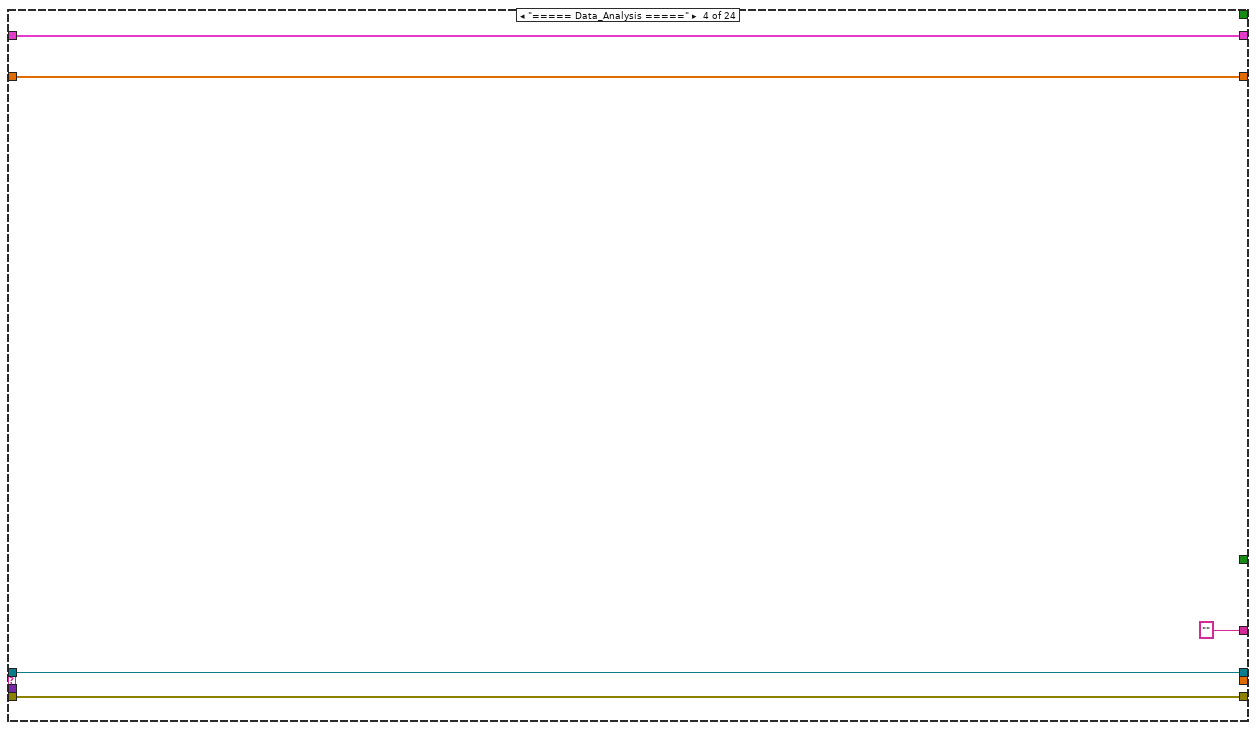
[diagram p6: hidden frame]
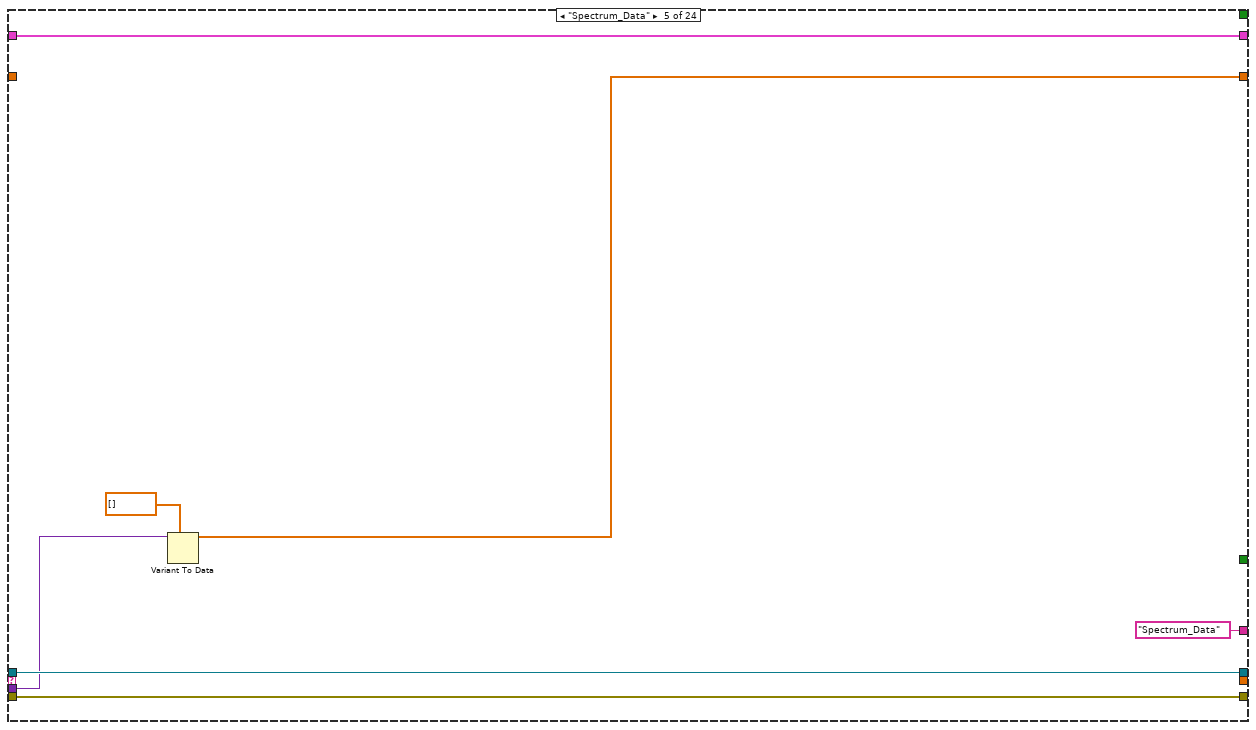
[diagram p7: hidden frame]
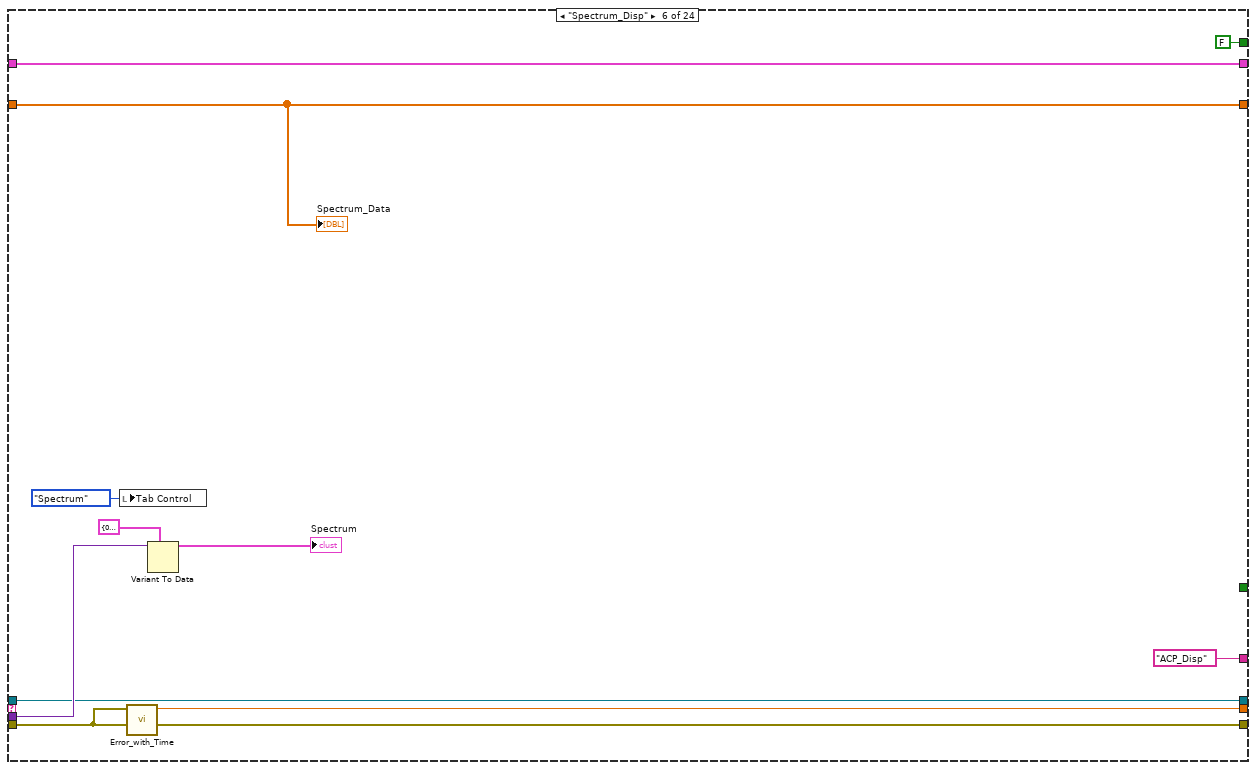
[diagram p8: hidden frame]
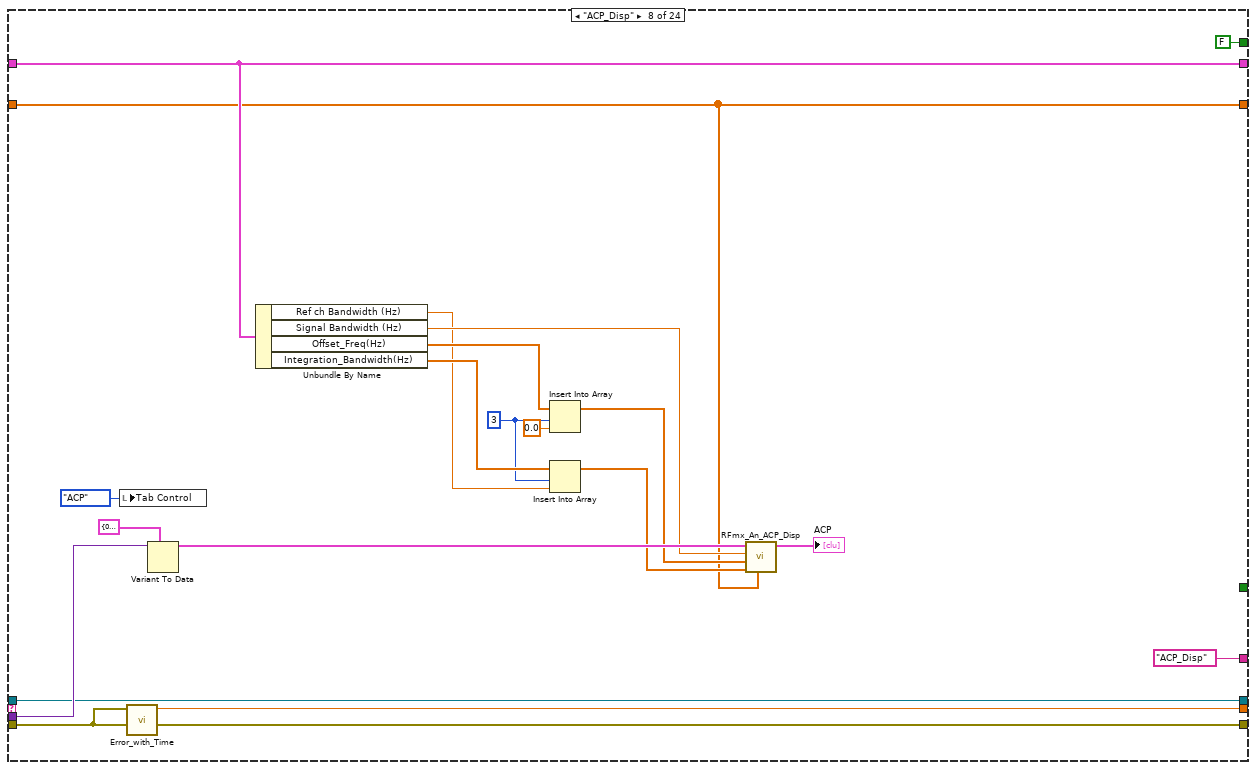
[diagram p9: hidden frame]
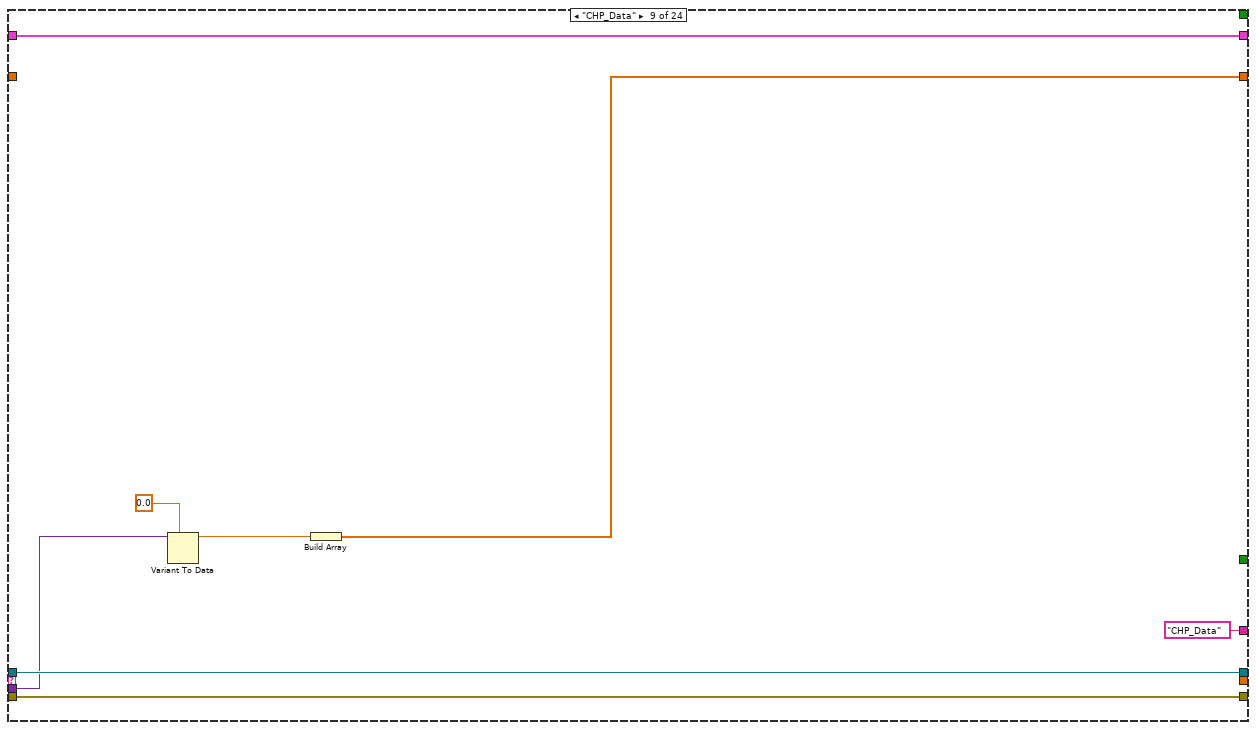
[diagram p10: hidden frame]
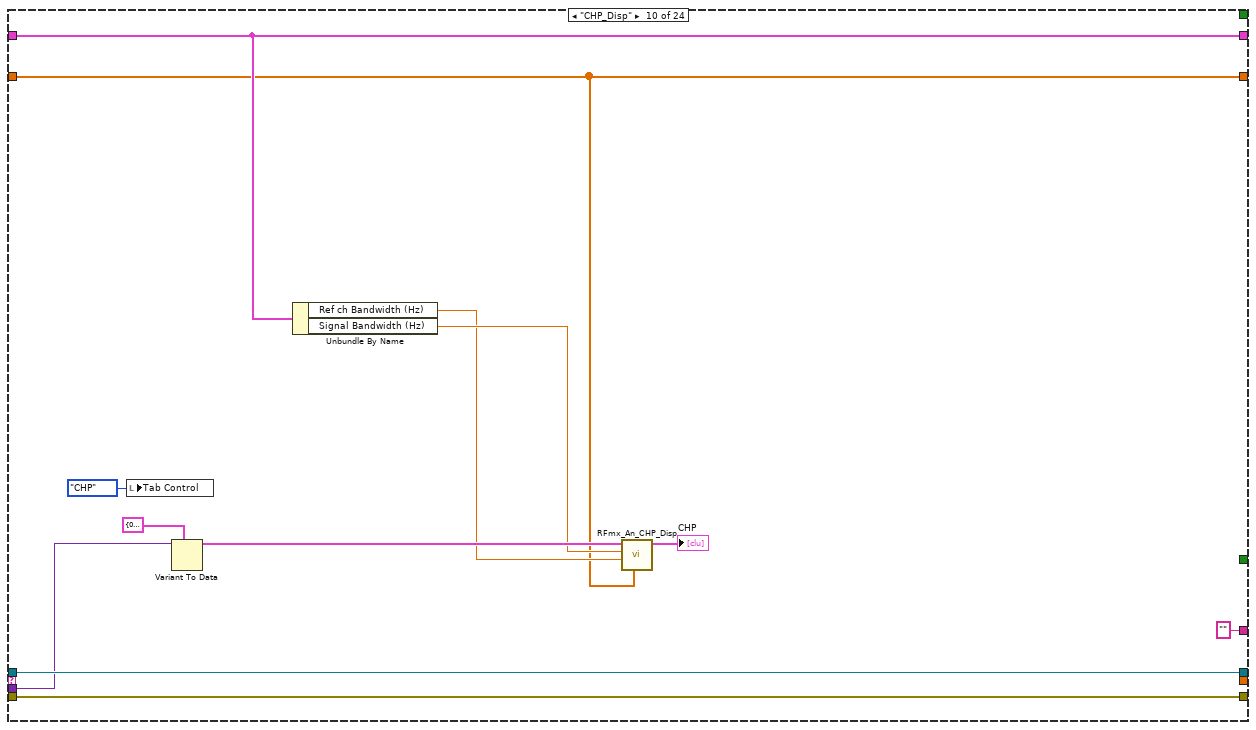
[diagram p11: hidden frame]
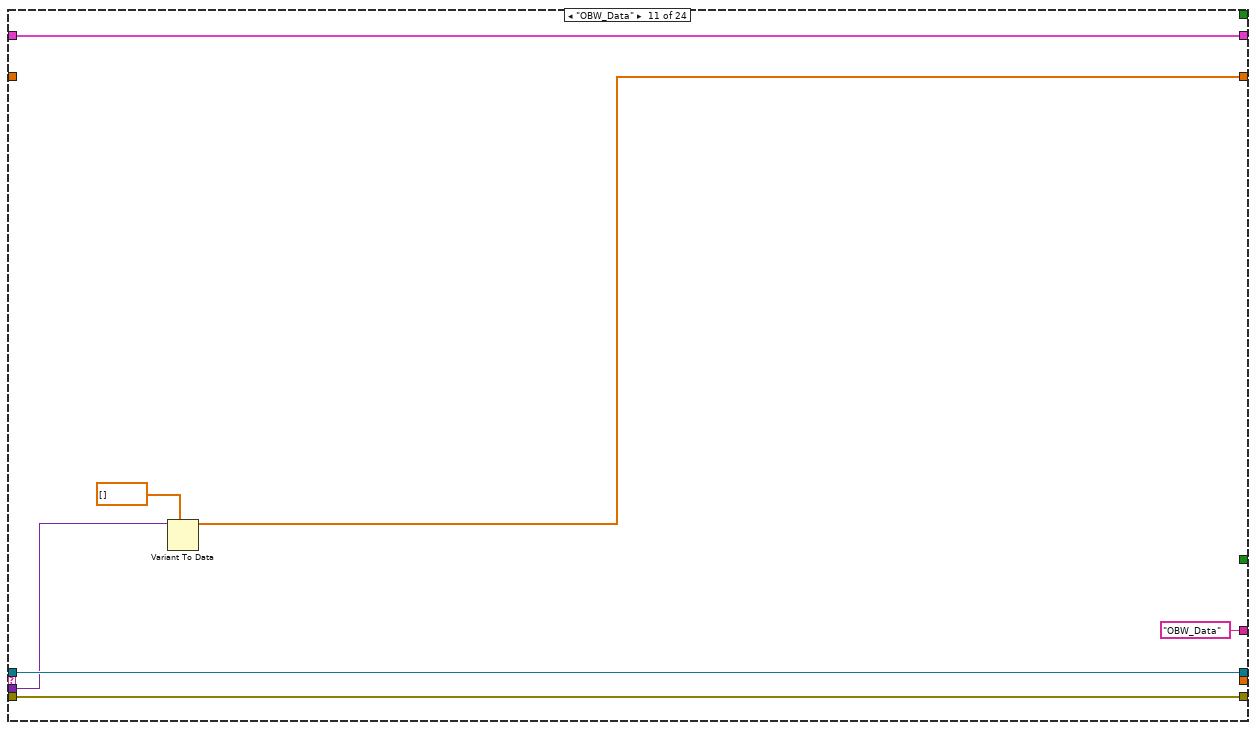
[diagram p12: hidden frame]
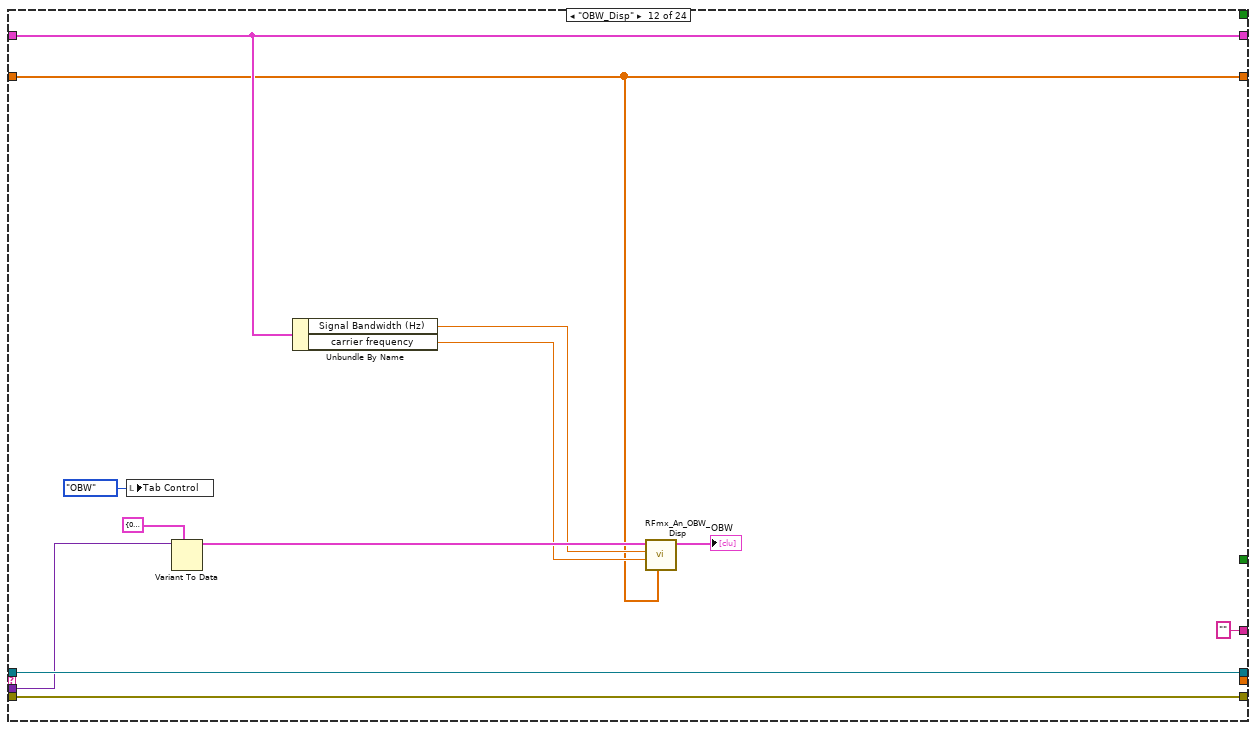
[diagram p13: hidden frame]
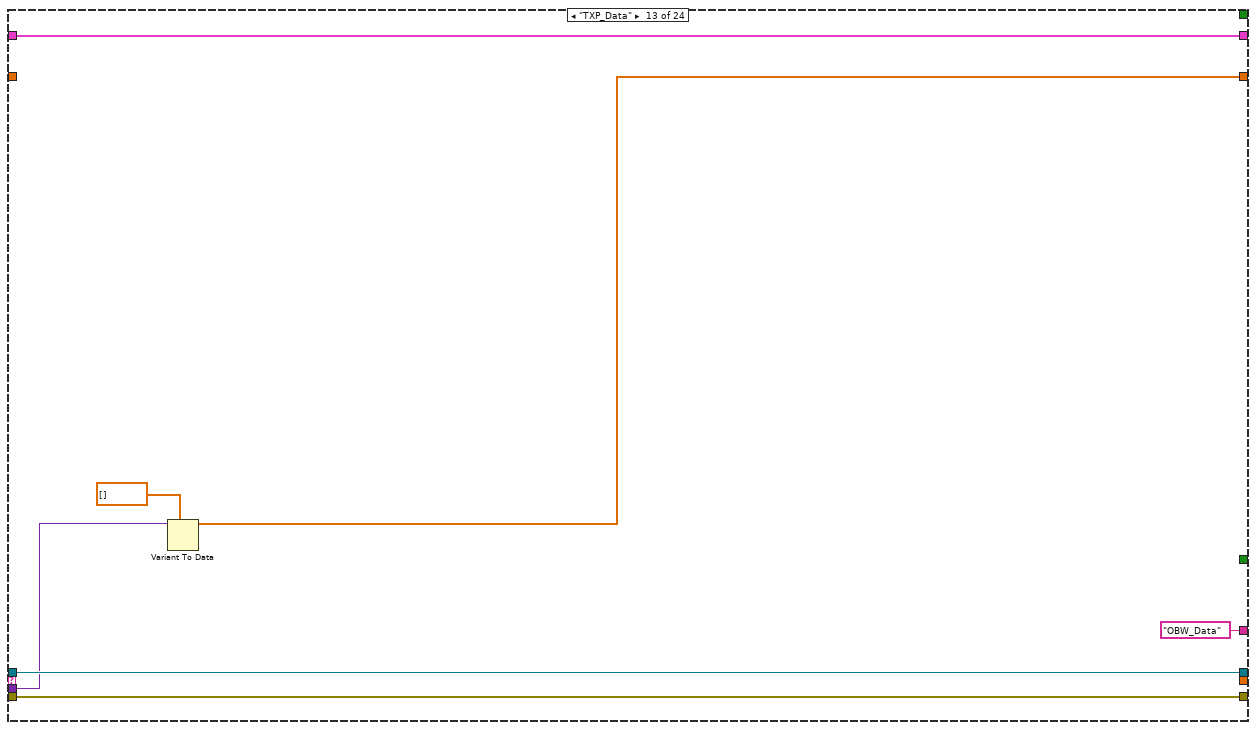
[diagram p14: hidden frame]
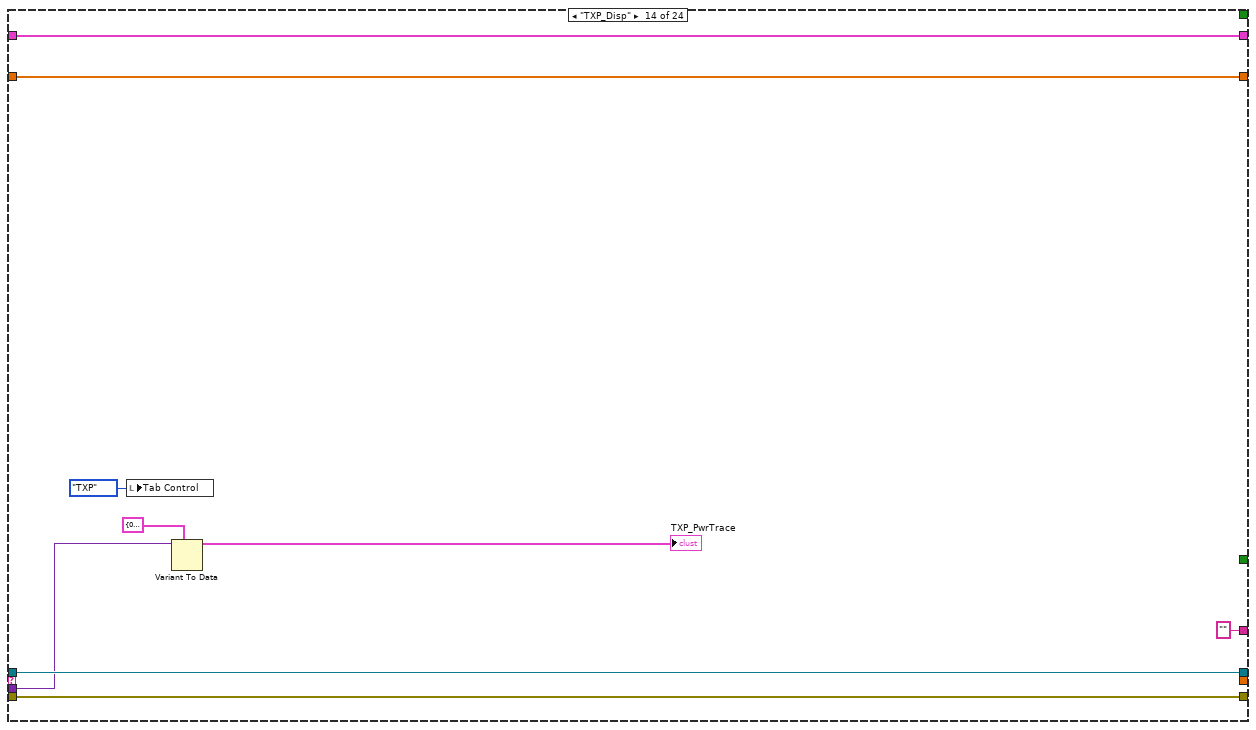
[diagram p15: hidden frame]
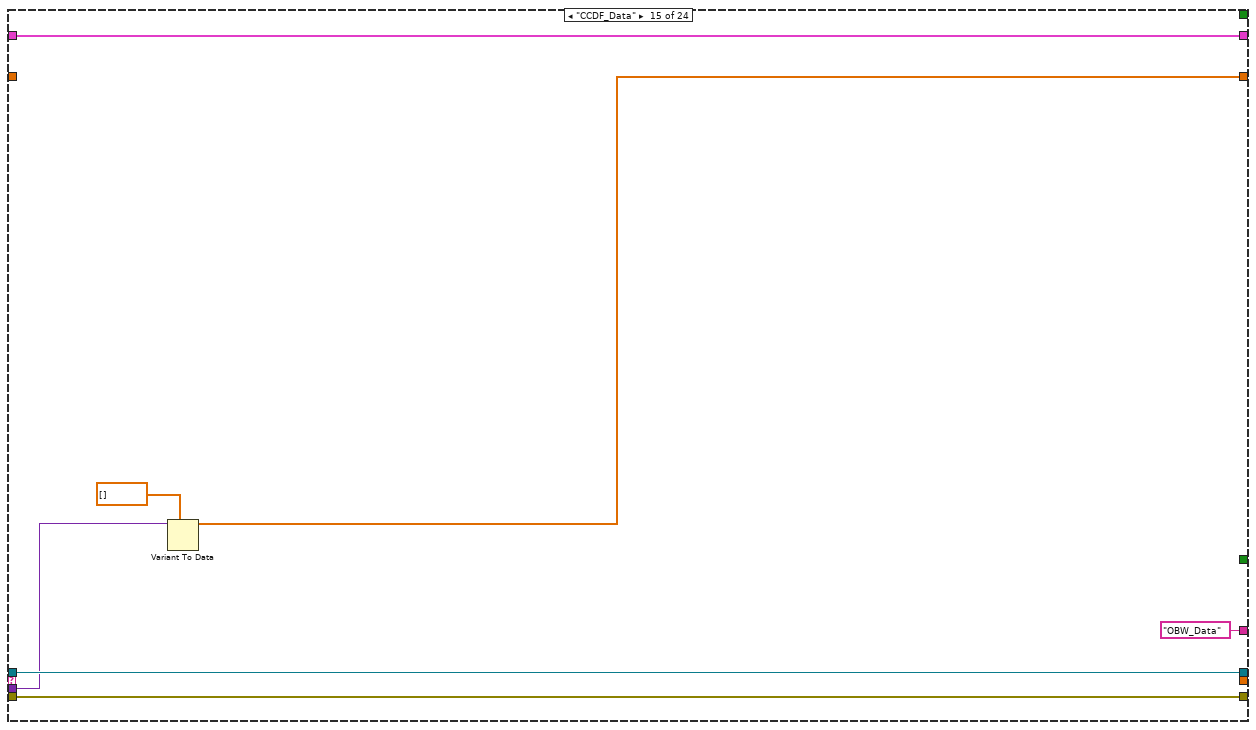
[diagram p16: hidden frame]
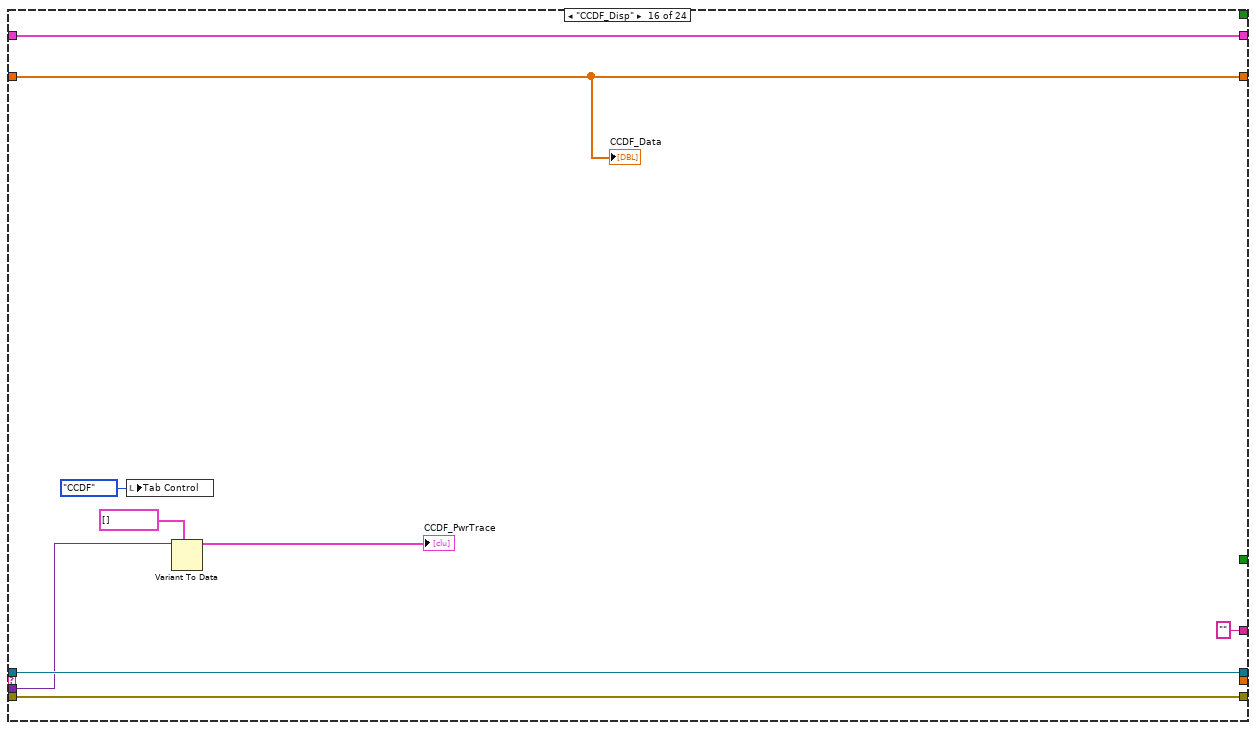
[diagram p17: hidden frame]
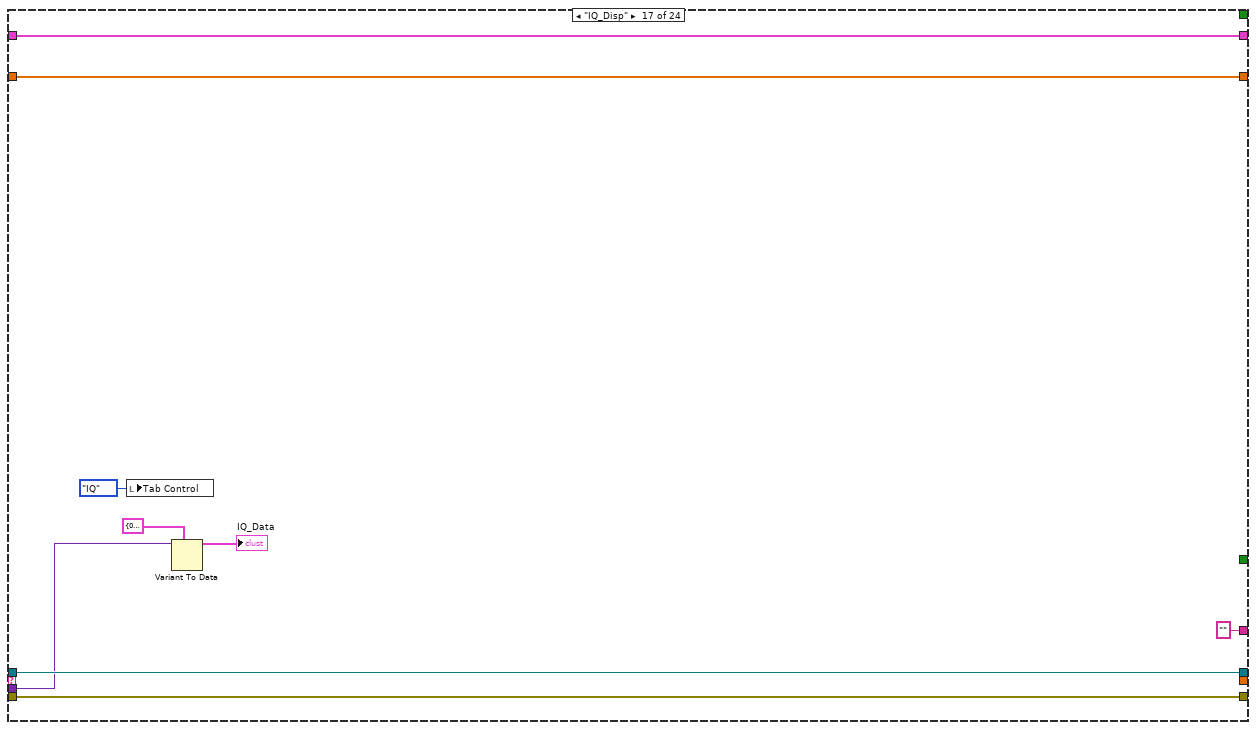
[diagram p18: hidden frame]
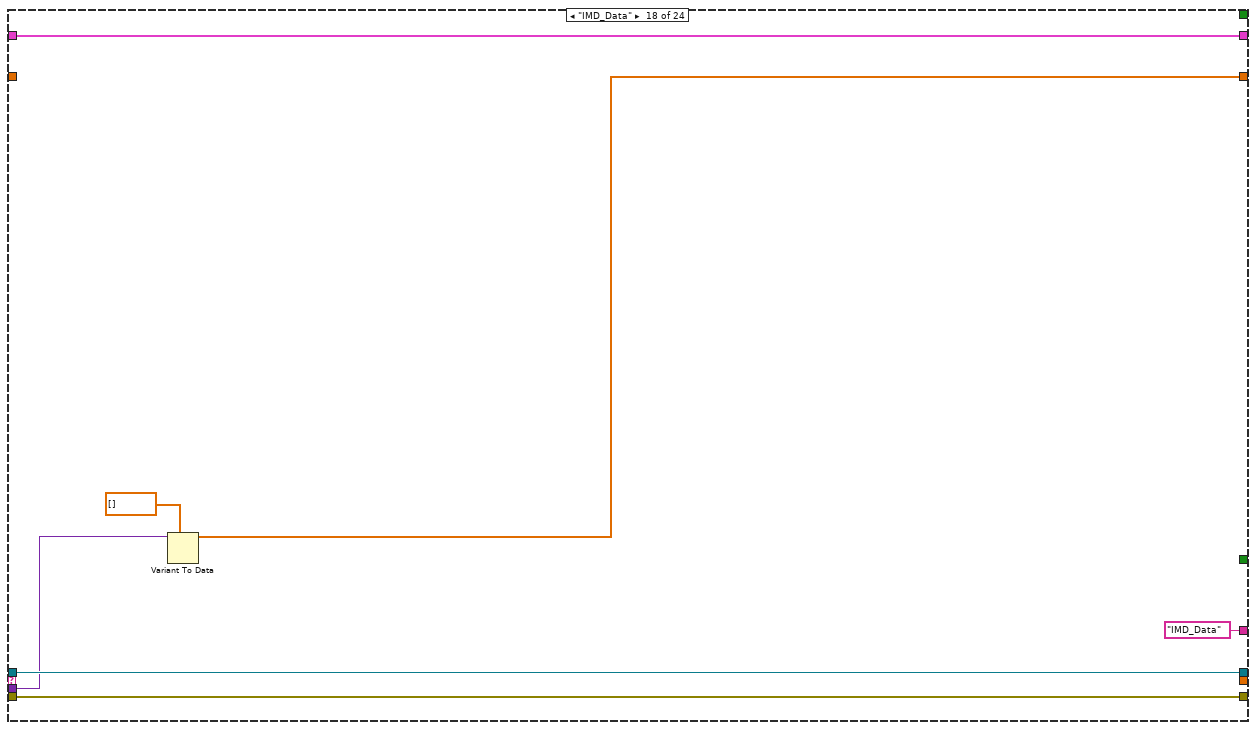
[diagram p19: hidden frame]
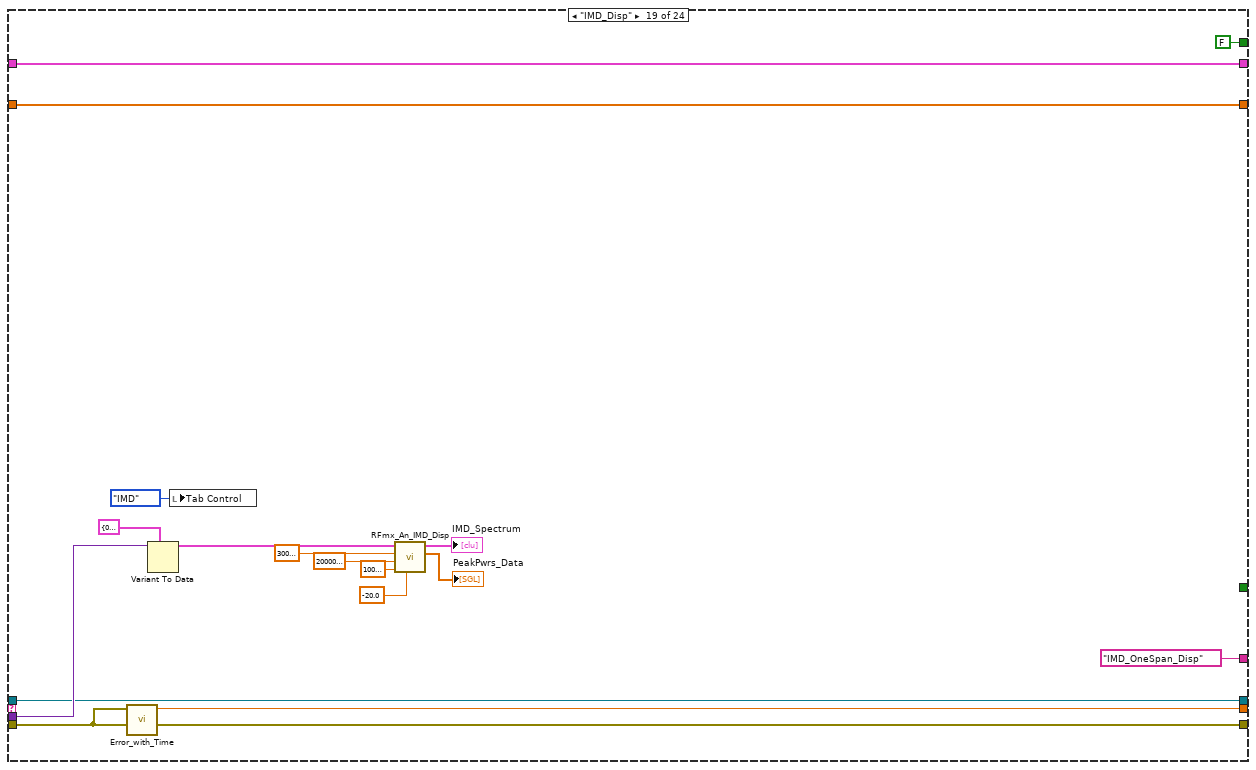
[diagram p20: hidden frame]
diagram:
  n1 = Unbundle By Name("Message_Queues") -> ("SysLog"=w3:refnum<queue>, "RFmx_Data"=w5:refnum<queue>)
  n2 = while {
    tunnel: "error in (no error)" -> [w27]
    tunnel: [w21] -> w6
    tunnel: w5 -> [w22]
    tunnel: w3 -> [w16]
    shift-right: [w11] -> _
    shift-left: "Analysis_Parameters" -> [w13]
    shift-right: [w8] -> _
    shift-left: dbl[] [] -> [w10]
    stop <- w15 stop-if-true
    # "RFmx Analysis Loop"
    n3 = call "DeQueue_Message.vi"("error in (no error)"=w27, "Message_Queue"=w22) -> ("error out"=w23:errorcluster, "Message Data"=w25:variant, "Message"=w26:string, "Dup_Message_Queue"=w24:refnum<queue>)  [unwired: 6 in]
    n4 = case "Main_Operation" shown="\"ACP_Data\"" w26 {
      tunnel: w25 -> [_ _ w57 _ w65 w80 w83 w107 w111 w122 w130 w142 w149 w158 w165 w175 w184 w190 w211 w214 w233 w236 w252 _]
      tunnel: w24 -> [w42 w49 w53 w60 w67 w79 w85 w106 w113 w127 w132 w146 w151 w162 w167 w178 w187 w192 w210 w216 w232 w238 w251 w258]
      tunnel: w23 -> [w44 w48 w54 w62 w68 w78 w86 w105 w114 w126 w133 w145 w152 w161 w168 w177 w186 w193 w209 w217 w231 w239 w250 w255]
      tunnel: [_ _ _ _ _ _ _ _ _ _ _ _ _ _ _ _ _ _ _ _ _ _ _ TRUE] -> w15
      tunnel: [w44 w48 w54 w62 w68 w78 w86 w105 w114 w126 w133 w145 w152 w161 w168 w177 w186 w193 w209 w217 w231 w239 w250 w255] -> w19
      tunnel: ["" ("Message") "" ("Message") "Update_Parameters" ("Message") "" ("Message") "Spectrum_Data" ("Message") "ACP_Disp" "ACP_Data" ("Message") "ACP_Disp" "CHP_Data" ("Message") "" ("Message") "OBW_Data" ("Message") "" ("Message") "OBW_Data" ("Message") "" ("Message") "OBW_Data" ("Message") "" ("Message") "" ("Message") "IMD_Data" ("Message") "IMD_OneSpan_Disp" "SFDR_Data" ("Message") "IMD_OneSpan_Disp" "Harmonics_Data" ("Message") "Harmonics_Disp" "RFSG_Exit" ("Message")] -> w20
      tunnel: [_ _ _ _ _ w77 _ w104 _ _ _ _ _ _ _ _ _ _ w208 _ w230 _ w249 w256] -> w18
      tunnel: [w42 w49 w53 w60 w67 w79 w85 w106 w113 w127 w132 w146 w151 w162 w167 w178 w187 w192 w210 w216 w232 w238 w251 w258] -> w17
      tunnel: [_ _ FALSE _ _ FALSE _ FALSE _ _ _ _ _ _ _ _ _ _ FALSE _ FALSE _ FALSE TRUE] -> w14
      tunnel: w13 -> [w41 w46 w56 w59 w69 w74 w87 w100 w115 w119 w134 w141 w153 w157 w169 w174 w183 w194 w205 w218 w227 w240 w246 w254]
      tunnel: [w41 w46 w55 w59 w69 w74 w87 w100 w115 w119 w134 w141 w153 w157 w169 w174 w183 w194 w205 w218 w227 w240 w246 w254] -> w12
      tunnel: w10 -> [w40 w45 w50 w58 _ w70 _ w88 _ w116 _ w135 _ w155 _ w171 w181 _ w203 _ w225 _ w241 w253]
      tunnel: [w40 w45 w50 w58 w63 w70 w81 w88 w108 w116 w128 w135 w147 w155 w163 w171 w181 w188 w203 w212 w225 w234 w241 w253] -> w9
      frame "Nothing", Default {
      }
      frame "===== Setting =====" {
      }
      frame "Update_Parameters" {
        n5 = Variant To Data(type=w56, Variant=w57) -> (data=w55:T2)  [unwired: 1 in, 1 out]
      }
      frame "===== Data_Analysis =====" {
      }
      frame "Spectrum_Data" {
        n6 = Variant To Data(type=dbl[] [], Variant=w65) -> (data=w63:dbl[])  [unwired: 1 in, 1 out]
      }
      frame "Spectrum_Disp" {
        n7 = local write "Tab Control"(RFmx_An_Disp_Ctrl."Spectrum" ("Tab Control")) -> ()
        n8 = call "Error_with_Time.vi"("error in (no error)"=w78) -> ("relative seconds"=w77:dbl)  [unwired: 10 in]
        n9 = Variant To Data(type=cluster{"x0":dbl, "dx":dbl, "y":sgl[]} {"x0"=0.0, "dx"=0.0, "y"=[]} ("Spectrum (dBm or dBm/Hz)"), Variant=w80) -> (data=→"Spectrum":cluster{"x0":dbl, "dx":dbl, "y":sgl[]})  [unwired: 1 in, 1 out]
        "Spectrum_Data" <- w70
      }
      frame "ACP_Data" {
        n10 = Variant To Data(type=dbl[] [], Variant=w83) -> (data=w81:dbl[])  [unwired: 1 in, 1 out]
        "ACP_Data" <- w81
      }
      frame "ACP_Disp" {
        w95 = 3 ("index")
        n11 = local write "Tab Control"(RFmx_An_Disp_Ctrl."ACP" ("Tab Control")) -> ()
        n12 = call "Error_with_Time.vi"("error in (no error)"=w105) -> ("relative seconds"=w104:dbl)  [unwired: 10 in]
        n13 = Variant To Data(type=cluster{"x0":dbl, "dx":dbl, "y":sgl[]} {"x0"=0.0, "dx"=0.0, "y"=[]} ("Spectrum (dBm or dBm/Hz)"), Variant=w107) -> (data=w101:cluster{"x0":dbl, "dx":dbl, "y":sgl[]})  [unwired: 1 in, 1 out]
        n14 = Unbundle By Name(w100) -> ("Ref ch Bandwidth (Hz)"=w94:dbl, "Signal Bandwidth (Hz)"=w99:dbl, "Offset_Freq(Hz)"=w98:dbl[], "Integration_Bandwidth(Hz)"=w96:dbl[])
        n15 = Insert Into Array(array=w98, index=w95, new element=0.0 ("new element/subarray")) -> (w93:dbl[])
        n16 = Insert Into Array(array=w96, index=w95, new element=w94) -> (w92:dbl[])
        n17 = call "RFmx_An_ACP_Disp.vi"("ACP_Values"=w88, "Int_Bandwidth"=w92, "Offsets"=w93, "SignalBandwidth"=w99, "Input_Waveform"=w101) -> ("Waveform Graph 2"=→"ACP":cluster{"x0":dbl, "dx":dbl, "y":sgl[]}[])  [unwired: 6 in]
      }
      frame "CHP_Data" {
        n18 = Variant To Data(type=0.0, Variant=w111) -> (data=w110:dbl)  [unwired: 1 in, 1 out]
        n19 = Build Array(w110) -> (w108:dbl[])
      }
      frame "CHP_Disp" {
        n20 = local write "Tab Control"(RFmx_An_Disp_Ctrl."CHP" ("Tab Control")) -> ()
        n21 = Variant To Data(type=cluster{"x0":dbl, "dx":dbl, "y":sgl[]} {"x0"=0.0, "dx"=0.0, "y"=[]} ("Spectrum (dBm or dBm/Hz)"), Variant=w122) -> (data=w123:cluster{"x0":dbl, "dx":dbl, "y":sgl[]})  [unwired: 1 in, 1 out]
        n22 = Unbundle By Name(w119) -> ("Ref ch Bandwidth (Hz)"=w120:dbl, "Signal Bandwidth (Hz)"=w121:dbl)
        n23 = call "RFmx_An_CHP_Disp.vi"("CHP_Values"=w116, "Int_Bandwidth"=w120, "SignalBandwidth"=w121, "Input_Waveform"=w123) -> ("Waveform Graph 2"=→"CHP":cluster{"x0":dbl, "dx":dbl, "y":sgl[]}[])  [unwired: 7 in]
      }
      frame "OBW_Data" {
        n24 = Variant To Data(type=dbl[] [], Variant=w130) -> (data=w128:dbl[])  [unwired: 1 in, 1 out]
      }
      frame "OBW_Disp" {
        n25 = local write "Tab Control"(RFmx_An_Disp_Ctrl."OBW" ("Tab Control")) -> ()
        n26 = Variant To Data(type=cluster{"x0":dbl, "dx":dbl, "y":sgl[]} {"x0"=0.0, "dx"=0.0, "y"=[]} ("Spectrum (dBm or dBm/Hz)"), Variant=w142) -> (data=w138:cluster{"x0":dbl, "dx":dbl, "y":sgl[]})  [unwired: 1 in, 1 out]
        n27 = Unbundle By Name(w141) -> ("Signal Bandwidth (Hz)"=w137:dbl, "carrier frequency"=w136:dbl)
        n28 = call "RFmx_An_OBW_Disp.vi"("OBW_Values"=w135, "CarrierFrequency"=w136, "SignalBandwidth"=w137, "Input_Waveform"=w138) -> ("Waveform Graph 2"=→"OBW":cluster{"x0":dbl, "dx":dbl, "y":sgl[]}[])  [unwired: 7 in]
      }
      frame "TXP_Data" {
        n29 = Variant To Data(type=dbl[] [], Variant=w149) -> (data=w147:dbl[])  [unwired: 1 in, 1 out]
      }
      frame "TXP_Disp" {
        n30 = local write "Tab Control"(RFmx_An_Disp_Ctrl."TXP" ("Tab Control")) -> ()
        n31 = Variant To Data(type=cluster{"x0":dbl, "dx":dbl, "y":sgl[]} {"x0"=0.0, "dx"=0.0, "y"=[]} ("Spectrum (dBm or dBm/Hz)"), Variant=w158) -> (data=→"TXP_PwrTrace":cluster{"x0":dbl, "dx":dbl, "y":sgl[]})  [unwired: 1 in, 1 out]
      }
      frame "CCDF_Data" {
        n32 = Variant To Data(type=dbl[] [], Variant=w165) -> (data=w163:dbl[])  [unwired: 1 in, 1 out]
      }
      frame "CCDF_Disp" {
        n33 = local write "Tab Control"(RFmx_An_Disp_Ctrl."CCDF" ("Tab Control")) -> ()
        n34 = Variant To Data(type=cluster{"x0":dbl, "dx":dbl, "y":sgl[]}[] [] ("appended array"), Variant=w175) -> (data=→"CCDF_PwrTrace":cluster{"x0":dbl, "dx":dbl, "y":sgl[]}[])  [unwired: 1 in, 1 out]
        "CCDF_Data" <- w171
      }
      frame "IQ_Disp" {
        n35 = local write "Tab Control"(RFmx_An_Disp_Ctrl."IQ" ("Tab Control")) -> ()
        n36 = Variant To Data(type=cluster{"t0":dbl, "dt":dbl, "Y":csg[]} {"t0"=0.0, "dt"=0.0, "Y"=[]} ("Data"), Variant=w184) -> (data=→"IQ_Data":cluster{"t0":dbl, "dt":dbl, "Y":csg[]})  [unwired: 1 in, 1 out]
      }
      frame "IMD_Data" {
        n37 = Variant To Data(type=dbl[] [], Variant=w190) -> (data=w188:dbl[])  [unwired: 1 in, 1 out]
      }
      frame "IMD_Disp" {
        n38 = call "Error_with_Time.vi"("error in (no error)"=w209) -> ("relative seconds"=w208:dbl)  [unwired: 10 in]
        n39 = Variant To Data(type=cluster{"x0":dbl, "dx":dbl, "y":sgl[]} {"x0"=0.0, "dx"=0.0, "y"=[]} ("Spectrum (dBm or dBm/Hz)"), Variant=w211) -> (data=w202:cluster{"x0":dbl, "dx":dbl, "y":sgl[]})  [unwired: 1 in, 1 out]
        n40 = local write "Tab Control"(RFmx_An_Disp_Ctrl."IMD" ("Tab Control")) -> ()
        n41 = call "RFmx_An_IMD_Disp.vi"("Target_Pwr(dBm)"=-20.0, "Int_Bandwidth(Hz)"=1000000.0, "Signal_Bandwidth(Hz)"=20000000.0, "Tone_Spacing(Hz)"=3000000.0, "IMD_Spectrum_in"=w202) -> ("PeakPwrs_Data"=→"PeakPwrs_Data":sgl[], "IMD_Spectrum_Out"=→"IMD_Spectrum":cluster{"x0":dbl, "dx":dbl, "y":sgl[]}[])  [unwired: 5 in]
      }
      frame "SFDR_Data" {
        n42 = Variant To Data(type=dbl[] [], Variant=w214) -> (data=w212:dbl[])  [unwired: 1 in, 1 out]
      }
      frame "SFDR_Disp" {
        n43 = call "Error_with_Time.vi"("error in (no error)"=w231) -> ("relative seconds"=w230:dbl)  [unwired: 10 in]
        n44 = Variant To Data(type=cluster{"x0":dbl, "dx":dbl, "y":sgl[]} {"x0"=0.0, "dx"=0.0, "y"=[]} ("Spectrum (dBm or dBm/Hz)"), Variant=w233) -> (data=w223:cluster{"x0":dbl, "dx":dbl, "y":sgl[]})  [unwired: 1 in, 1 out]
        n45 = local write "Tab Control"(RFmx_An_Disp_Ctrl."SFDR" ("Tab Control")) -> ()
        n46 = call "RFmx_An_SFDR_Disp.vi"("Int_Bandwidth(Hz)"=1000000.0, "Signal_Bandwidth(Hz)"=50000000.0, "IMD_Spectrum_in"=w223) -> ("PeakPwrs_Data"=→"PeakPwrs_Data 2":sgl[], "IMD_Spectrum_Out"=→"SFDR_Spectrum":cluster{"x0":dbl, "dx":dbl, "y":sgl[]}[])  [unwired: 7 in]
      }
      frame "Harmonics_Data" {
        n47 = Variant To Data(type=dbl[] [], Variant=w236) -> (data=w234:dbl[])  [unwired: 1 in, 1 out]
      }
      frame "Harmonics_Disp" {
        n48 = call "Error_with_Time.vi"("error in (no error)"=w250) -> ("relative seconds"=w249:dbl)  [unwired: 10 in]
        n49 = Variant To Data(type=cluster{"x0":dbl, "dx":dbl, "y":sgl[]}[] [], Variant=w252) -> (data=w242:cluster{"x0":dbl, "dx":dbl, "y":sgl[]}[])  [unwired: 1 in, 1 out]
        n50 = local write "Tab Control"(RFmx_An_Disp_Ctrl."Harmonics" ("Tab Control")) -> ()
        n51 = call "RFmx_An_Harms_Disp.vi"("Input_Spectrums"=w242) -> ("SFDR_Spectrum"=→"Harmonics_Spectrum":cluster{"x0":dbl, "dx":dbl, "y":sgl[]}[])  [unwired: 10 in]
        "PeakPwrs_Data 3" <- w241
      }
      frame "Exit" {
        n52 = call "Error_with_Time.vi"("error in (no error)"=w255) -> ("relative seconds"=w256:dbl)  [unwired: 10 in]
      }
    }
    n53 = case "Error_Handle" shown="False" w14 {
      tunnel: w19 -> [w30 w39]
      tunnel: [w30 w38] -> w21
      tunnel: w20 -> [_ w37]
      tunnel: w17 -> [_ w36]
      tunnel: w18 -> [_ w35]
      tunnel: w16 -> [_ w34]
      tunnel: w12 -> [w29 w32]
      tunnel: [w29 w32] -> w11
      tunnel: w9 -> [w28 w31]
      tunnel: [w28 w31] -> w8
      frame False {
      }
      frame True {
        n54 = call "SystemLog_with_Time.vi"("SysLog_Queue"=w34, "Message_in"=w37, "error in (no error)"=w39, "Send_Msg"="Exit", "Tick_in"=w35, "Worker_Queue"=w36) -> ("error out"=w38:errorcluster)  [unwired: 5 in]
      }
    }
  }
  "error out" <- w6
